vi "Meas Config Panel.vi"(8 "error in":errorcluster, 9 "force no GUI (False)":bool, 10 "always show setup (False)":bool, 11 "session in":T48={"adc"={"niScope"={"channel cfg"=[], "sessions"=[], "multi cards"=FALSE, "channels"=0, "type"=enum."n/a", "memory [B/chn]"=0, "ext. clock [Hz]"=0.0, "samples count"=0, "use streaming"=FALSE, "proc setup"={"packet size [smpl]"=0, "current timeout [s]"=0.0, "blk2blk timeout [s]"=0.0, "event time"=timestamp(0 s since 1904-01-01), "temp sampl T [s]"=0.0, "data queue"=refnum, "stop notifier"=refnum, "proc ref"=refnum}, "sample width [B]"=0, "ranges [V]"=[], "trigger setup"={"coupling"=1, "level [V]"=0.0, "slope"=0, "mode"=enum."Immediate"}, "fs [Hz]"=0.0, "bitres [bit]"=0}, "3458A"={"channels"=[], "sync unit"={"VISA"="", "type"=enum."Picotest U6200A"}, "awg unit"={"type"=enum."Agilent 331xxA to 332xxA", "VISA"="", "enable 10MHz ref"=FALSE}, "sync mode"=enum."MASTER-SLAVE, MASTER clocked by TIMER", "streaming mode"=FALSE, "idn mode"=enum."Auto", "sampling mode"=enum."DCV", "Ts [s]"=0.0, "sample memory [B]"=0, "proc setup"={"channel id"=0, "packet size [smpl]"=0, "current timeout [s]"=0.0, "blk2blk timeout [s]"=0.0, "event time"=timestamp(0 s since 1904-01-01), "stop notifier"=refnum, "data queues"=[], "proc refs"=[], "bus semaphore"=refnum}, "sample size [B]"=0, "sample count"=0, "aux data"={"channel id"=0, "valid?"=[], "gain [V]"=[], "timestamp [s]"=[], "Ts [s]"=0.0, "abs timestamp"=timestamp(0 s since 1904-01-01), "t [deg C]"=[]}, "ranges [V]"=[], "aperture [s]"=0.0, "LEVEL trigger"={"edge"=enum."POS", "level [V]"=0.0, "coupling"=enum."DC"}, "trigger mode"=enum."AUTO", "measure temp.?"=FALSE, "disp mesages"=[], "shared bus?"=FALSE, "disable display?"=FALSE, "aper mode"=enum."Manual", "aper rules"=[]}, "dsdll"={"dsdll"={"dsdll path"=path "", "dsdll handle"=[], "output devices"=[], "capture devices"=[]}, "channels"=0, "device id"=0, "channel idns"=[], "proc setup"={"packet size [smpl]"=0, "current timeout [s]"=0.0, "blk2blk timeout [s]"=0.0, "event time"=timestamp(0 s since 1904-01-01), "data queue"=refnum, "stop notifier"=refnum, "proc ref"=refnum}, "samples count"=0, "fs [Hz]"=0.0}, "type"=enum."niScope", "channel idn str"=[], "aux instr idn str"=[], "modified?"=FALSE, "simadc"={"channels"=[], "range [V]"=0.0, "Ts step [s]"=0.0, "time [s]"=0.0, "fs [Hz]"=0.0, "count"=0, "smpl offset"=0, "set count"=0, "bit res"=0}, "force rst?"=FALSE, "exit mode"=enum."Immediate reset", "exit dly"=0.0, "exit tmr"=timestamp(0 s since 1904-01-01), "busy?"=FALSE, "accessed?"=FALSE, "QuADC session"={"channel cfg"=[], "sessions"=[], "multi cards"=FALSE, "channels"=0, "type"=enum."n/a", "memory [B/chn]"=0, "ext. clock [Hz]"=0.0, "samples count"=0, "use streaming"=FALSE, "proc setup"={"packet size [smpl]"=0, "current timeout [s]"=0.0, "blk2blk timeout [s]"=0.0, "event time"=timestamp(0 s since 1904-01-01), "temp sampl T [s]"=0.0, "data queue"=refnum, "stop notifier"=refnum, "proc ref"=refnum}, "sample width [B]"=0, "ranges [V]"=[], "trigger setup"={"coupling"=1, "level [V]"=0.0, "slope"=0, "mode"=enum."Immediate"}, "fs [Hz]"=0.0, "bitres [bit]"=0}}, "sequence"=[], "sequence setup"={"group setups"=[], "average cycles"=0, "range mode"=enum."Keep defaults", "fs mode"=enum."Frequency", "rng even"=0.0, "rng odd"=0.0, "folder"=path "", "name base"="", "meas id"=0, "settle [s]"=0.0}, "golpi"=refnum, "processing setup"={"mode"=enum."Raw", "call after avgs?"=FALSE, "calculate?"=FALSE, "raw mode"={"command"="", "result mode"=enum."Display console output (only Octave)", "res variable"=""}, "QWTB"={"QWTB path"=path "", "alg filter path"="", "alg ids"=[], "alg parameters"=[], "parsed parameters"=[], "selected alg id"="", "selected unc mode"=enum."None", "qwtb mcc"=100, "qwtb timeout"=90, "qwtb covg"=95.0, "qwtb ofs"=0, "qwtb lim data"=0, "multicore"={"jobs folder"=path "", "cores"=0, "max jobs"=0, "mode"=enum."Singlecore"}, "unc once?"=FALSE}}, "corrections"={"transducers"={"channels"=[], "last path"=path ""}, "digitizer"={"last path"=path "", "channel paths"=[], "channel idns"=[], "correction name"="", "channel names"=[], "folders to copy"=[], "channel valid"=[], "correction path"=path "", "correction rel path"="", "rel folders to copy"=[]}}, "assist cfg"={"P"=0, "Q"=0, "rel shift"=0.0, "ref freq"=0.0, "min fs"=0.0, "max fs tol"=0.0, "min int"=0.0, "max int"=0.0, "max err"=0.0, "max timeout"=0.0}} {"corrections"."transducers"."channels"."Phase index" min=1 step=1; "adc"."QuADC session"."trigger setup"."level [V]" format="%.2f"; "adc"."QuADC session"."trigger setup"."coupling" items=["AC"=0, "DC"=1, "HF Reject"=3, "LF Reject"=4, "AC Plus HF Reject"=1001]; "adc"."QuADC session"."channel cfg"."Clock fr. (Hz)" min=0.0 format="%#_9p"; "adc"."QuADC session"."channel cfg"."Number of JJ" min=1; "adc"."QuADC session"."channel cfg"."Range [Vpk]" min=0.0; "adc"."QuADC session"."channel cfg"."Channel" min=0; "adc"."3458A"."channels"."Range [Vpk]" min=0.0; "adc"."niScope"."trigger setup"."level [V]" format="%.2f"; "adc"."niScope"."trigger setup"."coupling" items=["AC"=0, "DC"=1, "HF Reject"=3, "LF Reject"=4, "AC Plus HF Reject"=1001]; "adc"."niScope"."channel cfg"."Range [Vpk]" min=0.0; "adc"."niScope"."channel cfg"."Channel" min=0}) -> (0 "error out":errorcluster, 2 "canceled?":bool, 3 "session out":T48={"adc"={"niScope"={"channel cfg"=[], "sessions"=[], "multi cards"=FALSE, "channels"=0, "type"=enum."n/a", "memory [B/chn]"=0, "ext. clock [Hz]"=0.0, "samples count"=0, "use streaming"=FALSE, "proc setup"={"packet size [smpl]"=0, "current timeout [s]"=0.0, "blk2blk timeout [s]"=0.0, "event time"=timestamp(0 s since 1904-01-01), "temp sampl T [s]"=0.0, "data queue"=refnum, "stop notifier"=refnum, "proc ref"=refnum}, "sample width [B]"=0, "ranges [V]"=[], "trigger setup"={"coupling"=1, "level [V]"=0.0, "slope"=0, "mode"=enum."Immediate"}, "fs [Hz]"=0.0, "bitres [bit]"=0}, "3458A"={"channels"=[], "sync unit"={"VISA"="", "type"=enum."Picotest U6200A"}, "awg unit"={"type"=enum."Agilent 331xxA to 332xxA", "VISA"="", "enable 10MHz ref"=FALSE}, "sync mode"=enum."MASTER-SLAVE, MASTER clocked by TIMER", "streaming mode"=FALSE, "idn mode"=enum."Auto", "sampling mode"=enum."DCV", "Ts [s]"=0.0, "sample memory [B]"=0, "proc setup"={"channel id"=0, "packet size [smpl]"=0, "current timeout [s]"=0.0, "blk2blk timeout [s]"=0.0, "event time"=timestamp(0 s since 1904-01-01), "stop notifier"=refnum, "data queues"=[], "proc refs"=[], "bus semaphore"=refnum}, "sample size [B]"=0, "sample count"=0, "aux data"={"channel id"=0, "valid?"=[], "gain [V]"=[], "timestamp [s]"=[], "Ts [s]"=0.0, "abs timestamp"=timestamp(0 s since 1904-01-01), "t [deg C]"=[]}, "ranges [V]"=[], "aperture [s]"=0.0, "LEVEL trigger"={"edge"=enum."POS", "level [V]"=0.0, "coupling"=enum."DC"}, "trigger mode"=enum."AUTO", "measure temp.?"=FALSE, "disp mesages"=[], "shared bus?"=FALSE, "disable display?"=FALSE, "aper mode"=enum."Manual", "aper rules"=[]}, "dsdll"={"dsdll"={"dsdll path"=path "", "dsdll handle"=[], "output devices"=[], "capture devices"=[]}, "channels"=0, "device id"=0, "channel idns"=[], "proc setup"={"packet size [smpl]"=0, "current timeout [s]"=0.0, "blk2blk timeout [s]"=0.0, "event time"=timestamp(0 s since 1904-01-01), "data queue"=refnum, "stop notifier"=refnum, "proc ref"=refnum}, "samples count"=0, "fs [Hz]"=0.0}, "type"=enum."niScope", "channel idn str"=[], "aux instr idn str"=[], "modified?"=FALSE, "simadc"={"channels"=[], "range [V]"=0.0, "Ts step [s]"=0.0, "time [s]"=0.0, "fs [Hz]"=0.0, "count"=0, "smpl offset"=0, "set count"=0, "bit res"=0}, "force rst?"=FALSE, "exit mode"=enum."Immediate reset", "exit dly"=0.0, "exit tmr"=timestamp(0 s since 1904-01-01), "busy?"=FALSE, "accessed?"=FALSE, "QuADC session"={"channel cfg"=[], "sessions"=[], "multi cards"=FALSE, "channels"=0, "type"=enum."n/a", "memory [B/chn]"=0, "ext. clock [Hz]"=0.0, "samples count"=0, "use streaming"=FALSE, "proc setup"={"packet size [smpl]"=0, "current timeout [s]"=0.0, "blk2blk timeout [s]"=0.0, "event time"=timestamp(0 s since 1904-01-01), "temp sampl T [s]"=0.0, "data queue"=refnum, "stop notifier"=refnum, "proc ref"=refnum}, "sample width [B]"=0, "ranges [V]"=[], "trigger setup"={"coupling"=1, "level [V]"=0.0, "slope"=0, "mode"=enum."Immediate"}, "fs [Hz]"=0.0, "bitres [bit]"=0}}, "sequence"=[], "sequence setup"={"group setups"=[], "average cycles"=0, "range mode"=enum."Keep defaults", "fs mode"=enum."Frequency", "rng even"=0.0, "rng odd"=0.0, "folder"=path "", "name base"="", "meas id"=0, "settle [s]"=0.0}, "golpi"=refnum, "processing setup"={"mode"=enum."Raw", "call after avgs?"=FALSE, "calculate?"=FALSE, "raw mode"={"command"="", "result mode"=enum."Display console output (only Octave)", "res variable"=""}, "QWTB"={"QWTB path"=path "", "alg filter path"="", "alg ids"=[], "alg parameters"=[], "parsed parameters"=[], "selected alg id"="", "selected unc mode"=enum."None", "qwtb mcc"=100, "qwtb timeout"=90, "qwtb covg"=95.0, "qwtb ofs"=0, "qwtb lim data"=0, "multicore"={"jobs folder"=path "", "cores"=0, "max jobs"=0, "mode"=enum."Singlecore"}, "unc once?"=FALSE}}, "corrections"={"transducers"={"channels"=[], "last path"=path ""}, "digitizer"={"last path"=path "", "channel paths"=[], "channel idns"=[], "correction name"="", "channel names"=[], "folders to copy"=[], "channel valid"=[], "correction path"=path "", "correction rel path"="", "rel folders to copy"=[]}}, "assist cfg"={"P"=0, "Q"=0, "rel shift"=0.0, "ref freq"=0.0, "min fs"=0.0, "max fs tol"=0.0, "min int"=0.0, "max int"=0.0, "max err"=0.0, "max timeout"=0.0}} {"corrections"."transducers"."channels"."Phase index" min=1 step=1; "adc"."QuADC session"."trigger setup"."level [V]" format="%.2f"; "adc"."QuADC session"."trigger setup"."coupling" items=["AC"=0, "DC"=1, "HF Reject"=3, "LF Reject"=4, "AC Plus HF Reject"=1001]; "adc"."QuADC session"."channel cfg"."Clock fr. (Hz)" min=0.0 format="%#_9p"; "adc"."QuADC session"."channel cfg"."Number of JJ" min=1; "adc"."QuADC session"."channel cfg"."Range [Vpk]" min=0.0; "adc"."QuADC session"."channel cfg"."Channel" min=0; "adc"."3458A"."channels"."Range [Vpk]" min=0.0; "adc"."niScope"."trigger setup"."level [V]" format="%.2f"; "adc"."niScope"."trigger setup"."coupling" items=["AC"=0, "DC"=1, "HF Reject"=3, "LF Reject"=4, "AC Plus HF Reject"=1001]; "adc"."niScope"."channel cfg"."Range [Vpk]" min=0.0; "adc"."niScope"."channel cfg"."Channel" min=0})   [LabVIEW 2013]
doc: "New measurement configuration panel."
uses:
  Meas Session.ctl
  adc/ADC Session.ctl
  drivers/niScope/niScope Session.ctl
  drivers/niScope/niScope Virtual Channel Config.ctl
  drivers/niScope/niScope Virtual Channel Mode.ctl
  drivers/niScope/niScope Virtual Channel Input Z.ctl
  drivers/niScope/niScope Virtual Channel Coupling.ctl
  drivers/niScope/niScope Type.ctl
  drivers/niScope/niScope Digitizing Process Options.ctl
  drivers/niScope/niScope Data Packet.ctl
  drivers/niScope/niScope Trigger Setup.ctl
  <instrlib>/niScope/Controls/niScope trigger coupling.ctl
  <instrlib>/niScope/Controls/niScope trigger slope.ctl
  drivers/DMM/3458A Digitizer Session.ctl
  drivers/DMM/3458A Virtual Channel Config.ctl
  drivers/Counter/Counter Session.ctl
  drivers/Counter/Counter Type.ctl
  drivers/AWG/AWG Session.ctl
  drivers/AWG/AWG Type.ctl
  drivers/DMM/3458A Sync Mode.ctl
  drivers/DMM/3458A Idn Mode.ctl
  drivers/DMM/3458A Digitizing Low Levels/Configure/Sampling Mode.ctl
  drivers/DMM/3458A Digitizing Process Options.ctl
  drivers/DMM/3458A Data Packet.ctl
  drivers/DMM/3458A Aux Record Data.ctl
  drivers/DMM/3458A Digitizing Low Levels/Configure/Level Setup.ctl
  drivers/DMM/3458A Digitizing Low Levels/Configure/First Sample Trigger.ctl
  drivers/DMM/3458A Aperture Selection Mode.ctl
  drivers/dsdll/DSDLL Session.ctl
  drivers/dsdll/dsdll.lvlibp/dsdll_instance.ctl
  drivers/dsdll/dsdll.lvlibp/dsdll_device_record.ctl
  drivers/dsdll/DSDLL Process Config.ctl
  drivers/dsdll/DSDLL Data Packet.ctl
  adc/ADC Type.ctl
  drivers/simulated_adc/SimAdc Config.ctl
  drivers/simulated_adc/SimAdc Channel Cfg.ctl
  adc/ADC On Close Action.ctl
  drivers/Quatsch_driver/QuADCDriver/QuADC Session.ctl
  drivers/Quatsch_driver/QuADCDriver/QuADC Virtual Channel Config.ctl
  drivers/Quatsch_driver/QuADCDriver/QuADC Virtual Channel Mode.ctl
  drivers/Quatsch_driver/QuADCDriver/QuADC Virtual Channel Input Z.ctl
  drivers/Quatsch_driver/QuADCDriver/QuADC Virtual Channel Coupling.ctl
  drivers/Quatsch_driver/QuADCDriver/QuADC Type.ctl
  drivers/Quatsch_driver/QuADCDriver/QuADC Digitizing Process Options.ctl
  drivers/Quatsch_driver/QuADCDriver/QuADC Data Packet.ctl
  drivers/Quatsch_driver/QuADCDriver/QuADC Trigger Setup.ctl
  Meas Sequence Item.ctl
  Meas Sampling Configuration.ctl
  adc/ADC Trig Config.ctl
  adc/ADC Trig Mode Source.ctl
  adc/ADC Trig Coupling.ctl
  adc/ADC Trig Slope.ctl
  processing/QWTB/Meas Proc QWTB Algorithm Parameter Data.ctl
  Meas Sequence Configuration.ctl
  Meas Range Mode.ctl
  Meas Sampling Rate Mode.ctl
  octave/golpi/mpc/golpi_session_ref.ctl
  octave/golpi/mpc/golpi_session.ctl
  octave/golpi/GOLPI Library.lvlibp/Public/GOLPI reference Type Def.ctl
  octave/golpi/GOLPI Library.lvlibp/LV Process source distribution/Pipe Handle.ctl
  processing/Meas Process Config.ctl
  processing/Meas Process Mode.ctl
  processing/Meas Process Raw Config.ctl
  processing/Meas Process Raw Result Mode.ctl
  processing/QWTB/Meas Proc QWTB Setup.ctl
  processing/QWTB/Meas Proc QWTB Uncertainty Mode.ctl
  processing/QWTB/Meas Proc QWTB Multicore Setup.ctl
  processing/QWTB/Meas Proc QWTB Multicore Type.ctl
  Corrections/Corr Setup.ctl
  Corrections/Corr Tranducer Item.ctl
  Corrections/Corr Digitizers.ctl
  Assist/Assist Panel Setup.ctl
  varilib/SGUI Assign References Mode.ctl
  other/GUI Panel Control Action.ctl
  adc/ADC Capabilities Parameters.ctl
  varilib/SGUI Set Multiple Reals By Label.vi
  varilib/SGUI Set Single Real By Label.vi
  varilib/SGUI Set Single Integer By Label.vi
  varilib/varilib.lvlib
  drivers/niScope/niScope Virtual Digitizer.lvlib
  drivers/DMM/3458A Virtual Digitizer.lvlib
  drivers/Counter/Counter.lvlib
  drivers/AWG/AWG.lvlib
  drivers/DMM/3458A Digitizing Low Levels/3458A Digitizing Low Levels.lvlib
  drivers/dsdll/dsdll.lvlibp
  drivers/dsdll/DSDLL Virtual Digitizer.lvlib
  octave/golpi/GOLPI Library.lvlibp/LV Process source distribution/LV Process library.lvlib
  octave/golpi/GOLPI Library.lvlibp
  octave/golpi/mpc/GOLPI Multi Process.lvlib
  drivers/Quatsch_driver/QuADCDriver/QuADC Virtual Digitizer.lvlib
panel:
  in  "rep delay":dbl caption="Repetition settling [s]"
  in  "btn assist":bool
  in  "smpl time":dbl caption="Meas. time [s]"
  out "smpl time max":dbl caption="Max. time [s]" format="%#_6p"
  out "meas full":path caption="Full measurement base path preview"
  in  "meas id":i32 caption="Measurement number" min=0 max=9999 step=1
  in  "btn proc":bool
  in  "calc result?":bool caption="Enable result calculation?"
  in  "meas name":string caption="Measurement name base"
  in  "data folder":path caption="Folder for measurements data files"
  in  "avg cycles":i32=1 caption="Repetition cycles"
  in  "range even":dbl
  in  "range odd":dbl caption="All ranges [V]"
  in  "range mode":T1 caption="Voltage range selection"
  out "smpl count max":dbl caption="Max. samples count" format="%#_6p"
  in  "smpl count":i64 caption="Samples count"
  out "aperture max":dbl caption="smpl rate min" format="%#_5p"
  out "aperture min":dbl caption="Aperture range [s]" format="%#_5p"
  out "smpl rate max":dbl caption="smpl rate min" format="%#_5p"
  out "smpl rate min":dbl caption="Sampling period range [s]" format="%#_5p"
  in  "trig coupling":T2 caption="Trigger coupling"
  in  "trig slope":T3 caption="Trigger slope"
  in  "trig level":dbl caption="Level [V]" format="%#_3p"
  in  "trig mode":T4 caption="Trigger mode"
  in  "aperture":dbl caption="Aperture [s]" format="%#_3p"
  out "adc":T5={"niScope"={"channel cfg"=[], "sessions"=[], "multi cards"=FALSE, "channels"=0, "type"=enum."n/a", "memory [B/chn]"=0, "ext. clock [Hz]"=0.0, "samples count"=0, "use streaming"=FALSE, "proc setup"={"packet size [smpl]"=0, "current timeout [s]"=0.0, "blk2blk timeout [s]"=0.0, "event time"=timestamp(0 s since 1904-01-01), "temp sampl T [s]"=0.0, "data queue"=refnum, "stop notifier"=refnum, "proc ref"=refnum}, "sample width [B]"=0, "ranges [V]"=[], "trigger setup"={"coupling"=1, "level [V]"=0.0, "slope"=0, "mode"=enum."Immediate"}, "fs [Hz]"=0.0, "bitres [bit]"=0}, "3458A"={"channels"=[], "sync unit"={"VISA"="", "type"=enum."Picotest U6200A"}, "awg unit"={"type"=enum."Agilent 331xxA to 332xxA", "VISA"="", "enable 10MHz ref"=FALSE}, "sync mode"=enum."MASTER-SLAVE, MASTER clocked by TIMER", "streaming mode"=FALSE, "idn mode"=enum."Auto", "sampling mode"=enum."DCV", "Ts [s]"=0.0, "sample memory [B]"=0, "proc setup"={"channel id"=0, "packet size [smpl]"=0, "current timeout [s]"=0.0, "blk2blk timeout [s]"=0.0, "event time"=timestamp(0 s since 1904-01-01), "stop notifier"=refnum, "data queues"=[], "proc refs"=[], "bus semaphore"=refnum}, "sample size [B]"=0, "sample count"=0, "aux data"={"channel id"=0, "valid?"=[], "gain [V]"=[], "timestamp [s]"=[], "Ts [s]"=0.0, "abs timestamp"=timestamp(0 s since 1904-01-01), "t [deg C]"=[]}, "ranges [V]"=[], "aperture [s]"=0.0, "LEVEL trigger"={"edge"=enum."POS", "level [V]"=0.0, "coupling"=enum."DC"}, "trigger mode"=enum."AUTO", "measure temp.?"=FALSE, "disp mesages"=[], "shared bus?"=FALSE, "disable display?"=FALSE, "aper mode"=enum."Manual", "aper rules"=[]}, "dsdll"={"dsdll"={"dsdll path"=path "", "dsdll handle"=[], "output devices"=[], "capture devices"=[]}, "channels"=0, "device id"=0, "channel idns"=[], "proc setup"={"packet size [smpl]"=0, "current timeout [s]"=0.0, "blk2blk timeout [s]"=0.0, "event time"=timestamp(0 s since 1904-01-01), "data queue"=refnum, "stop notifier"=refnum, "proc ref"=refnum}, "samples count"=0, "fs [Hz]"=0.0}, "type"=enum."niScope", "channel idn str"=[], "aux instr idn str"=[], "modified?"=FALSE, "simadc"={"channels"=[], "range [V]"=0.0, "Ts step [s]"=0.0, "time [s]"=0.0, "fs [Hz]"=0.0, "count"=0, "smpl offset"=0, "set count"=0, "bit res"=0}, "force rst?"=FALSE, "exit mode"=enum."Immediate reset", "exit dly"=0.0, "exit tmr"=timestamp(0 s since 1904-01-01), "busy?"=FALSE, "accessed?"=FALSE, "QuADC session"={"channel cfg"=[], "sessions"=[], "multi cards"=FALSE, "channels"=0, "type"=enum."n/a", "memory [B/chn]"=0, "ext. clock [Hz]"=0.0, "samples count"=0, "use streaming"=FALSE, "proc setup"={"packet size [smpl]"=0, "current timeout [s]"=0.0, "blk2blk timeout [s]"=0.0, "event time"=timestamp(0 s since 1904-01-01), "temp sampl T [s]"=0.0, "data queue"=refnum, "stop notifier"=refnum, "proc ref"=refnum}, "sample width [B]"=0, "ranges [V]"=[], "trigger setup"={"coupling"=1, "level [V]"=0.0, "slope"=0, "mode"=enum."Immediate"}, "fs [Hz]"=0.0, "bitres [bit]"=0}} {"QuADC session"."trigger setup"."level [V]" format="%.2f"; "QuADC session"."trigger setup"."coupling" items=["AC"=0, "DC"=1, "HF Reject"=3, "LF Reject"=4, "AC Plus HF Reject"=1001]; "QuADC session"."channel cfg"."Clock fr. (Hz)" min=0.0 format="%#_9p"; "QuADC session"."channel cfg"."Number of JJ" min=1; "QuADC session"."channel cfg"."Range [Vpk]" min=0.0; "QuADC session"."channel cfg"."Channel" min=0; "3458A"."channels"."Range [Vpk]" min=0.0; "niScope"."trigger setup"."level [V]" format="%.2f"; "niScope"."trigger setup"."coupling" items=["AC"=0, "DC"=1, "HF Reject"=3, "LF Reject"=4, "AC Plus HF Reject"=1001]; "niScope"."channel cfg"."Range [Vpk]" min=0.0; "niScope"."channel cfg"."Channel" min=0}
  in  "btn cancel":bool
  in  "btn ok":bool
  in  "fs mode":T47 caption="Sampling rate mode"
  in  "smpl rate":dbl caption="Sampling period [s]"
  # "Use following variables in the name base:\n  %id% - measurement number in format DDDD\n  %date% - date of the measurement YYYYMMDD\n  %time% - time of the measurement HH-MM-SS\nExample:\n  my_measurement_%id%"
  # "IP Address"
  # "."
  # "."
  # "."
  # ":"
  # "ADC:"
  # "IP Address"
  # "."
  # "."
  # "."
  # ":"
  # "ADC:"
  # "IP Address"
  # "."
  # "."
  # "."
  # ":"
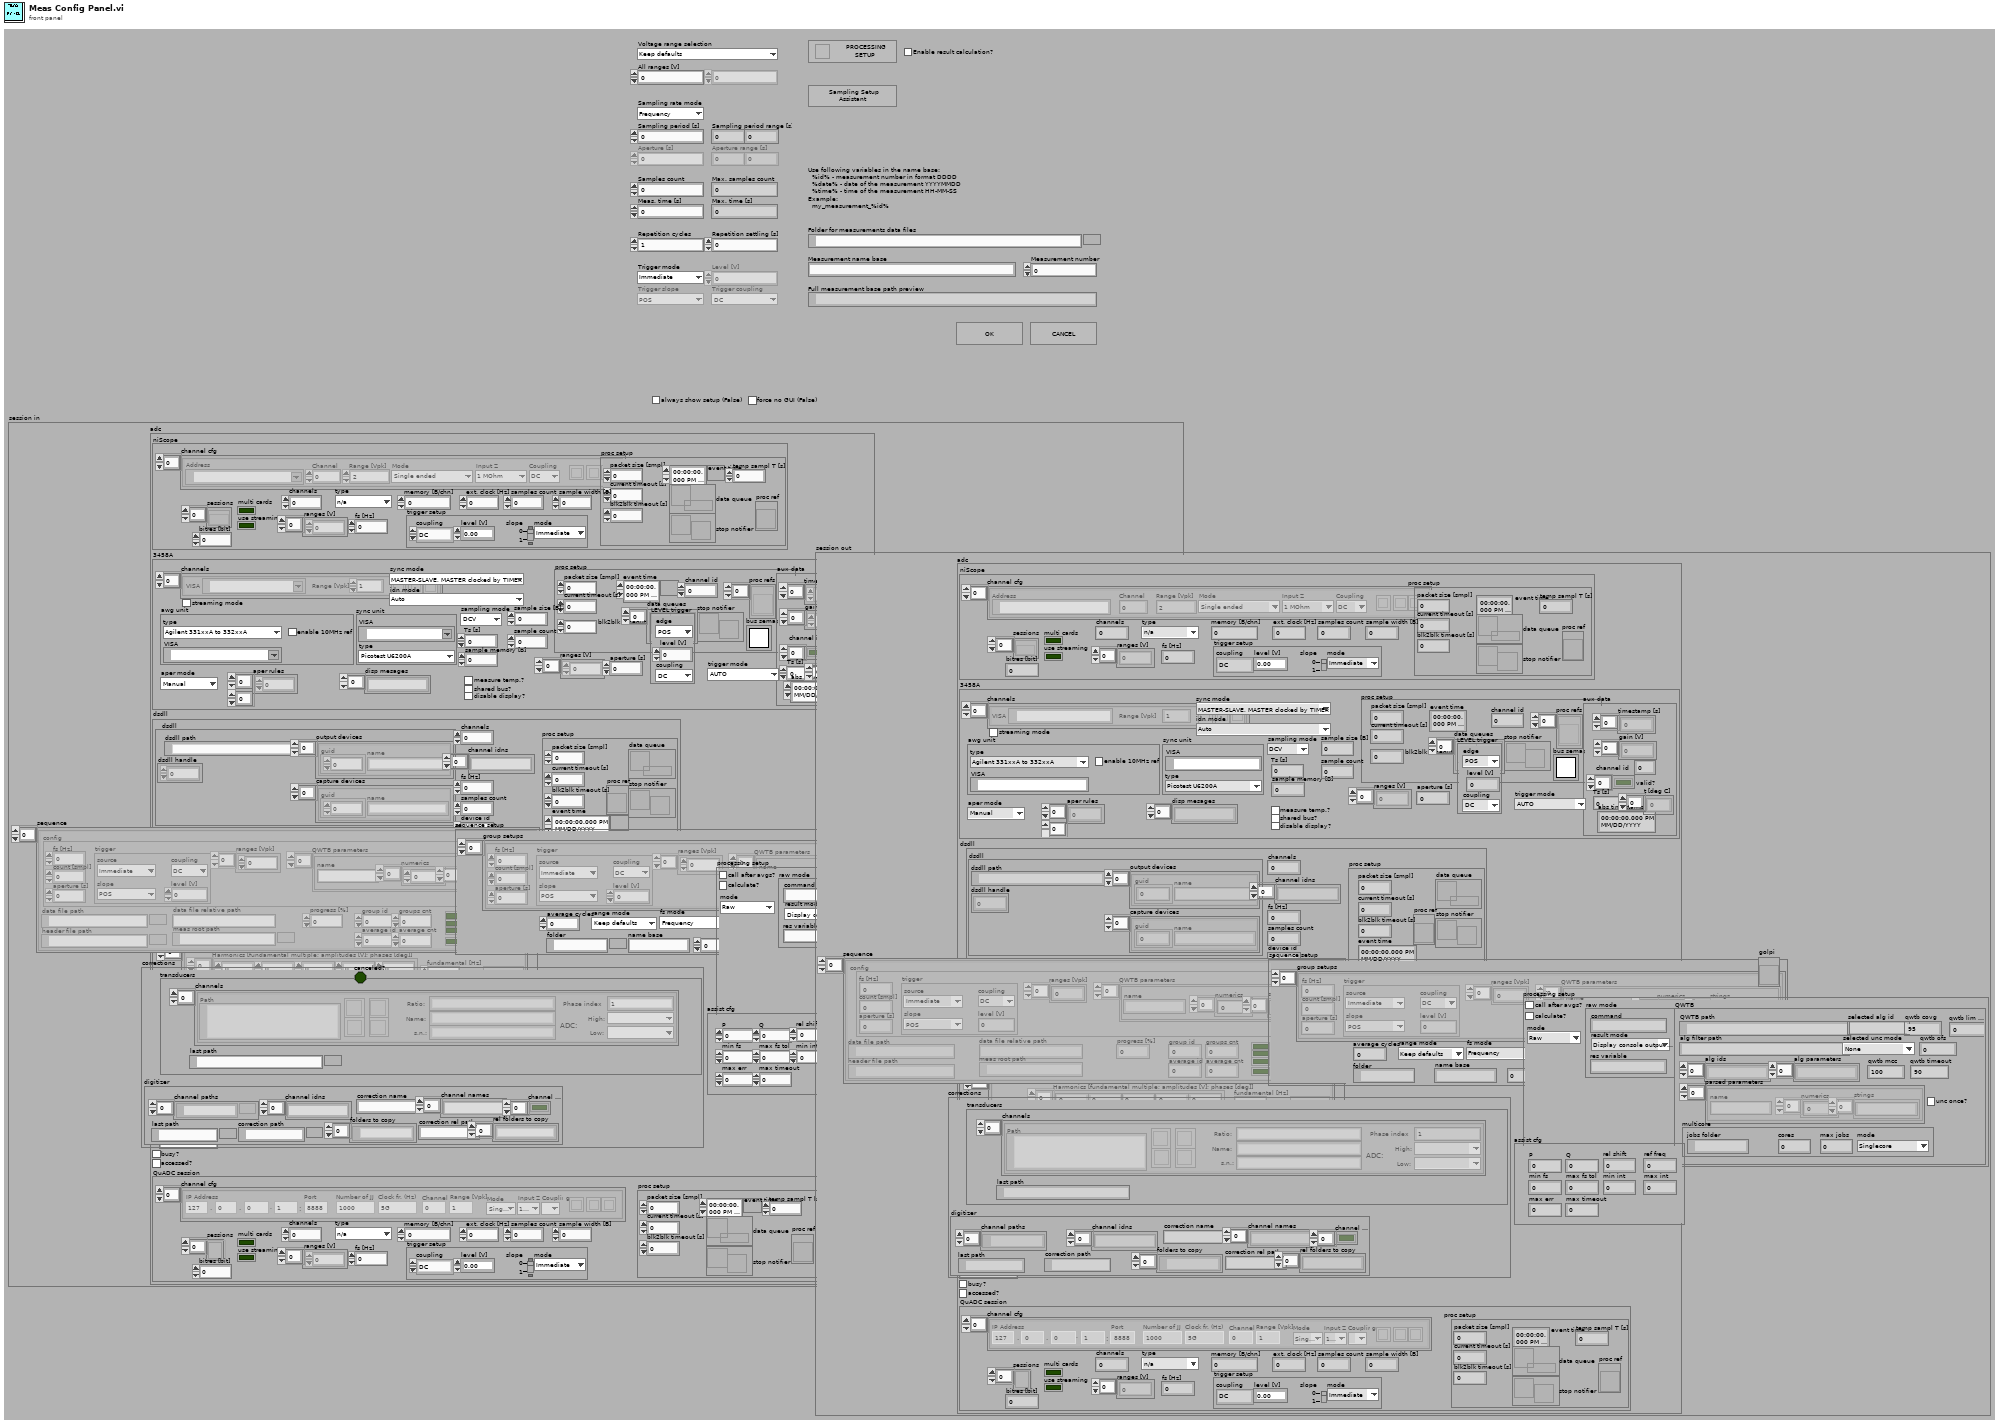
[diagram p1: front panel]
types:
  T1 = typedef "Meas Range Mode.ctl" = enum16{"Keep defaults", "Set All channels", "Set Odd and Even channels"}
  T2 = typedef "ADC Trig Coupling.ctl" = enum16{"DC", "AC"}
  T3 = typedef "ADC Trig Slope.ctl" = enum16{"POS", "NEG"}
  T4 = typedef "ADC Trig Mode Source.ctl" = enum16{"Immediate", "External", "Level"}
  T5 = typedef "ADC Session.ctl" = cluster{"niScope":T6, "3458A":T16, "dsdll":T31, "type":T35, "channel idn str":string[], "aux instr idn str":string[], "modified?":bool, "simadc":T36, "force rst?":bool, "exit mode":T38, "exit dly":dbl, "exit tmr":timestamp, "busy?":bool, "accessed?":bool, "QuADC session":T39}
  T6 = typedef "niScope Virtual Digitizer.lvlib/niScope Session.ctl" = cluster{"channel cfg":T7[], "sessions":refnum<k20>[], "multi cards":bool, "channels":i32, "type":T11, "memory [B/chn]":i32, "ext. clock [Hz]":dbl, "samples count":i64, "use streaming":bool, "proc setup":T12, "sample width [B]":i32, "ranges [V]":dbl[], "trigger setup":T13, "fs [Hz]":dbl, "bitres [bit]":i32}
  T7 = typedef "niScope Virtual Digitizer.lvlib/niScope Virtual Channel Config.ctl" = cluster{"Address":refnum<k15>, "Channel":i32, "Mode":T8, "Input Z":T9, "Coupling":T10, "Range [Vpk]":dbl, "btn clr":bool, "btn up":bool, "btn down":bool}
  T8 = typedef "niScope Virtual Digitizer.lvlib/niScope Virtual Channel Mode.ctl" = enum16{"Single ended", "Unbal. differential", "Differential"}
  T9 = typedef "niScope Virtual Digitizer.lvlib/niScope Virtual Channel Input Z.ctl" = enum16{"1 MOhm", "50 Ohm"}
  T10 = typedef "niScope Virtual Digitizer.lvlib/niScope Virtual Channel Coupling.ctl" = enum16{"AC", "DC", "GND"}
  T11 = typedef "niScope Virtual Digitizer.lvlib/niScope Type.ctl" = enum16{"n/a", "5922"}
  T12 = typedef "niScope Virtual Digitizer.lvlib/niScope Digitizing Process Options.ctl" = cluster{"packet size [smpl]":i64, "current timeout [s]":dbl, "blk2blk timeout [s]":dbl, "event time":timestamp, "temp sampl T [s]":dbl, "data queue":refnum<queue>, "stop notifier":refnum<notifier>, "proc ref":refnum<vi>}
  T13 = typedef "niScope Virtual Digitizer.lvlib/niScope Trigger Setup.ctl" = cluster{"coupling":T14, "level [V]":dbl, "slope":T15, "mode":enum16{"Immediate", "External", "Level"}}
  T14 = typedef "niScope trigger coupling.ctl" = u16
  T15 = typedef "niScope trigger slope.ctl" = i32
  T16 = typedef "3458A Virtual Digitizer.lvlib/3458A Digitizer Session.ctl" = cluster{"channels":T17[], "sync unit":T18, "awg unit":T20, "sync mode":T22, "streaming mode":bool, "idn mode":T23, "sampling mode":T24, "Ts [s]":dbl, "sample memory [B]":i32, "proc setup":T25, "sample size [B]":i32, "sample count":i32, "aux data":T27, "ranges [V]":dbl[], "aperture [s]":dbl, "LEVEL trigger":T28, "trigger mode":T29, "measure temp.?":bool, "disp mesages":string[], "shared bus?":bool, "disable display?":bool, "aper mode":T30, "aper rules":dbl[][]}
  T17 = typedef "3458A Virtual Digitizer.lvlib/3458A Virtual Channel Config.ctl" = cluster{"VISA":refnum<visa-resource-name>, "Range [Vpk]":dbl, "btn clr":bool, "btn up":bool, "btn down":bool}
  T18 = typedef "Counter.lvlib/Counter Session.ctl" = cluster{"VISA":refnum<visa-resource-name>, "type":T19}
  T19 = typedef "Counter.lvlib/Counter Type.ctl" = enum16{"Picotest U6200A", "dummy"}
  T20 = typedef "AWG.lvlib/AWG Session.ctl" = cluster{"type":T21, "VISA":refnum<visa-resource-name>, "enable 10MHz ref":bool}
  T21 = typedef "AWG.lvlib/AWG Type.ctl" = enum16{"Agilent 331xxA to 332xxA", "Agilent 335xxA to 336xxA", "Tektronix AFG3101C", "dummy"}
  T22 = typedef "3458A Virtual Digitizer.lvlib/3458A Sync Mode.ctl" = enum16{"MASTER-SLAVE, MASTER clocked by TIMER", "MASTER-SLAVE, MASTER clocked by AWG", "ALL clocked by AWG", "MASTER-SLAVE, ALL clocked by TIMER", "ALL clocked by AWG with DFLL"}
  T23 = typedef "3458A Virtual Digitizer.lvlib/3458A Idn Mode.ctl" = enum16{"Auto", "Sequential (chn A, chn B, ...)", "From calibration string"}
  T24 = typedef "3458A Virtual Digitizer.lvlib/3458A Digitizing Low Levels.lvlib/Sampling Mode.ctl" = enum16{"DCV", "DSDC", "DSAC"}
  T25 = typedef "3458A Virtual Digitizer.lvlib/3458A Digitizing Process Options.ctl" = cluster{"channel id":i32, "packet size [smpl]":i32, "current timeout [s]":dbl, "blk2blk timeout [s]":dbl, "event time":timestamp, "stop notifier":refnum<notifier>, "data queues":refnum<queue>[], "proc refs":refnum<vi>[], "bus semaphore":T26}
  T26 = typedef "Semaphore RefNum" = refnum<k1>
  T27 = typedef "3458A Virtual Digitizer.lvlib/3458A Aux Record Data.ctl" = cluster{"channel id":i32, "valid?":bool[], "gain [V]":dbl[], "timestamp [s]":dbl[], "Ts [s]":dbl, "abs timestamp":timestamp, "t [deg C]":dbl[]}
  T28 = typedef "3458A Virtual Digitizer.lvlib/3458A Digitizing Low Levels.lvlib/Level Setup.ctl" = cluster{"edge":enum16{"POS", "NEG"}, "level [V]":dbl, "coupling":enum16{"DC", "AC"}}
  T29 = typedef "3458A Virtual Digitizer.lvlib/3458A Digitizing Low Levels.lvlib/First Sample Trigger.ctl" = enum16{"AUTO", "EXT", "SYN", "SGL", "HOLD", "LEVEL"}
  T30 = typedef "3458A Virtual Digitizer.lvlib/3458A Aperture Selection Mode.ctl" = enum16{"Manual", "Maximum", "Table"}
  T31 = typedef "DSDLL Virtual Digitizer.lvlib/DSDLL Session.ctl" = cluster{"dsdll":T32, "channels":i32, "device id":i32, "channel idns":string[], "proc setup":T34, "samples count":i32, "fs [Hz]":dbl}
  T32 = typedef "dsdll.lvlibp/dsdll_instance.ctl" = cluster{"dsdll path":path, "dsdll handle":u8[], "output devices":T33[], "capture devices":T33[]}
  T33 = typedef "dsdll.lvlibp/dsdll_device_record.ctl" = cluster{"guid":u8[], "name":string}
  T34 = typedef "DSDLL Virtual Digitizer.lvlib/DSDLL Process Config.ctl" = cluster{"packet size [smpl]":i32, "current timeout [s]":dbl, "blk2blk timeout [s]":dbl, "event time":timestamp, "data queue":refnum<queue>, "stop notifier":refnum<notifier>, "proc ref":refnum<vi>}
  T35 = typedef "ADC Type.ctl" = enum16{"niScope", "3458A", "DirectSound DLL", "dummy", "QuADC"}
  T36 = typedef "SimAdc Config.ctl" = cluster{"channels":T37[], "range [V]":dbl, "Ts step [s]":dbl, "time [s]":dbl, "fs [Hz]":dbl, "count":i64, "smpl offset":i64, "set count":i64, "bit res":i32}
  T37 = typedef "SimAdc Channel Cfg.ctl" = cluster{"harmonics":dbl[][], "btn clear":bool, "noise":dbl, "fundamental [Hz]":dbl}
  T38 = typedef "ADC On Close Action.ctl" = enum16{"Immediate reset", "Delayed reset"}
  T39 = typedef "QuADC Virtual Digitizer.lvlib/QuADC Session.ctl" = cluster{"channel cfg":T40[], "sessions":refnum<k5>[], "multi cards":bool, "channels":i32, "type":T44, "memory [B/chn]":i32, "ext. clock [Hz]":dbl, "samples count":i64, "use streaming":bool, "proc setup":T45, "sample width [B]":i32, "ranges [V]":dbl[], "trigger setup":T46, "fs [Hz]":dbl, "bitres [bit]":i32}
  T40 = typedef "QuADC Virtual Digitizer.lvlib/QuADC Virtual Channel Config.ctl" = cluster{"Channel":i32, "Mode":T41, "Input Z":T42, "Coupling":T43, "Range [Vpk]":dbl, "btn clr":bool, "btn up":bool, "btn down":bool, "IP address A":u8, "IP address B":u8, "IP address C":u8, "IP address D":u8, "Port":u16, "Number of JJ":u32, "Clock fr. (Hz)":dbl}
  T41 = typedef "QuADC Virtual Digitizer.lvlib/QuADC Virtual Channel Mode.ctl" = enum16{"Single ended", "Unbal. differential", "Differential"}
  T42 = typedef "QuADC Virtual Digitizer.lvlib/QuADC Virtual Channel Input Z.ctl" = enum16{"1 MOhm", "50 Ohm"}
  T43 = typedef "QuADC Virtual Digitizer.lvlib/QuADC Virtual Channel Coupling.ctl" = enum16{"AC", "DC", "GND"}
  T44 = typedef "QuADC Virtual Digitizer.lvlib/QuADC Type.ctl" = enum16{"n/a", "v1"}
  T45 = typedef "QuADC Virtual Digitizer.lvlib/QuADC Digitizing Process Options.ctl" = cluster{"packet size [smpl]":i64, "current timeout [s]":dbl, "blk2blk timeout [s]":dbl, "event time":timestamp, "temp sampl T [s]":dbl, "data queue":refnum<queue>, "stop notifier":refnum<notifier>, "proc ref":refnum<vi>}
  T46 = typedef "QuADC Virtual Digitizer.lvlib/QuADC Trigger Setup.ctl" = cluster{"coupling":T14, "level [V]":dbl, "slope":T15, "mode":enum16{"Immediate", "External", "Level"}}
  T47 = typedef "Meas Sampling Rate Mode.ctl" = enum16{"Frequency", "Period"}
  T48 = typedef "Meas Session.ctl" = cluster{"adc":T5, "sequence":T49[], "sequence setup":T53, "golpi":T54, "processing setup":T55, "corrections":T63, "assist cfg":T66}
  T49 = typedef "Meas Sequence Item.ctl" = cluster{"config":T50, "data file path":path, "header file path":path, "group id":i32, "average id":i32, "group done?":bool, "adc modified?":bool, "source modified?":bool, "progress [%]":dbl, "groups cnt":i32, "average cnt":i32, "data file relative path":string, "meas root path":path, "calculate?":bool}
  T50 = typedef "Meas Sampling Configuration.ctl" = cluster{"fs [Hz]":dbl, "count [smpl]":i64, "aperture [s]":dbl, "trigger":T51, "ranges [Vpk]":dbl[], "QWTB parameters":T52[]}
  T51 = typedef "ADC Trig Config.ctl" = cluster{"source":T4, "level [V]":dbl, "coupling":T2, "slope":T3}
  T52 = typedef "Meas Proc QWTB Algorithm Parameter Data.ctl" = cluster{"name":string, "numerics":dbl[], "strings":string[]}
  T53 = typedef "Meas Sequence Configuration.ctl" = cluster{"group setups":T50[], "average cycles":i32, "range mode":T1, "fs mode":T47, "rng even":dbl, "rng odd":dbl, "folder":path, "name base":string, "meas id":i32, "settle [s]":dbl}
  T54 = typedef "GOLPI Multi Process.lvlib/golpi_session_ref.ctl" = refnum<vi>
  T55 = typedef "Meas Process Config.ctl" = cluster{"mode":T56, "call after avgs?":bool, "calculate?":bool, "raw mode":T57, "QWTB":T59}
  T56 = typedef "Meas Process Mode.ctl" = enum16{"Raw", "QWTB"}
  T57 = typedef "Meas Process Raw Config.ctl" = cluster{"command":string, "result mode":T58, "res variable":string}
  T58 = typedef "Meas Process Raw Result Mode.ctl" = enum16{"Display console output (only Octave)", "Display string variable", "Display result file %respath%"}
  T59 = typedef "Meas Proc QWTB Setup.ctl" = cluster{"QWTB path":path, "alg filter path":string, "alg ids":string[], "alg parameters":string[], "parsed parameters":T52[], "selected alg id":string, "selected unc mode":T60, "qwtb mcc":i32, "qwtb timeout":i32, "qwtb covg":dbl, "qwtb ofs":i64, "qwtb lim data":i64, "multicore":T61, "unc once?":bool}
  T60 = typedef "Meas Proc QWTB Uncertainty Mode.ctl" = enum16{"None", "GUF", "Monte Carlo"}
  T61 = typedef "Meas Proc QWTB Multicore Setup.ctl" = cluster{"jobs folder":path, "cores":i32, "max jobs":i32, "mode":T62}
  T62 = typedef "Meas Proc QWTB Multicore Type.ctl" = enum16{"Singlecore", "Multicore", "Multistation"}
  T63 = typedef "Corr Setup.ctl" = cluster{"transducers":cluster{"channels":T64[], "last path":path}, "digitizer":T65}
  T64 = typedef "Corr Tranducer Item.ctl" = cluster{"Path":path, "Ratio:":string, "Name:":string, "btn rem":bool, "btn up":bool, "btn down":bool, "s.n.:":string, "btn open":bool, "ratio o/i":dbl, "chn hi":u16, "chn lo":u16, "Phase index":i32}
  T65 = typedef "Corr Digitizers.ctl" = cluster{"last path":path, "channel paths":path[], "channel idns":string[], "correction name":string, "channel names":string[], "folders to copy":path[], "channel valid":bool[], "correction path":path, "correction rel path":string, "rel folders to copy":string[]}
  T66 = typedef "Assist Panel Setup.ctl" = cluster{"P":i32, "Q":i32, "rel shift":dbl, "ref freq":dbl, "min fs":dbl, "max fs tol":dbl, "min int":dbl, "max int":dbl, "max err":dbl, "max timeout":dbl}
  T67 = typedef "GUI Panel Control Action.ctl" = enum16{"Open panel", "Close panel", "Bring To Front"}
  T68 = typedef "varilib.lvlib/SGUI Assign References Mode.ctl" = enum16{"Add to stack", "Overwrite", "Release last", "Release ID"}
  T69 = typedef "ADC Capabilities Parameters.ctl" = cluster{"fs [Hz]":dbl, "aperture [s]":dbl}
  T70 = typedef "ADC Capabilities.ctl" = cluster{"max samples count":i64, "max fs [Hz]":ext, "min fs [Hz]":ext, "Ts step [s]":ext, "max Ts [s]":ext, "min Ts [s]":ext, "allows streaming?":bool, "streaming on?":bool, "has level trig?":bool, "has ext trig?":bool, "has aperture?":bool, "aper min [s]":dbl, "aper max [s]":dbl, "channels count":i32, "has ranges?":bool, "has temperature?":bool, "has temperature log?":bool, "has selfcal?":bool, "fs step [Hz]":ext, "smpl rate step mode":T71}
  T71 = typedef "ADC Sampling Rate Step Mode.ctl" = enum16{"const period", "const frequency"}
  T72 = typedef "Assist Sampling Setup.ctl" = cluster{"fs [Hz]":ext, "N":i64, "error":dbl}
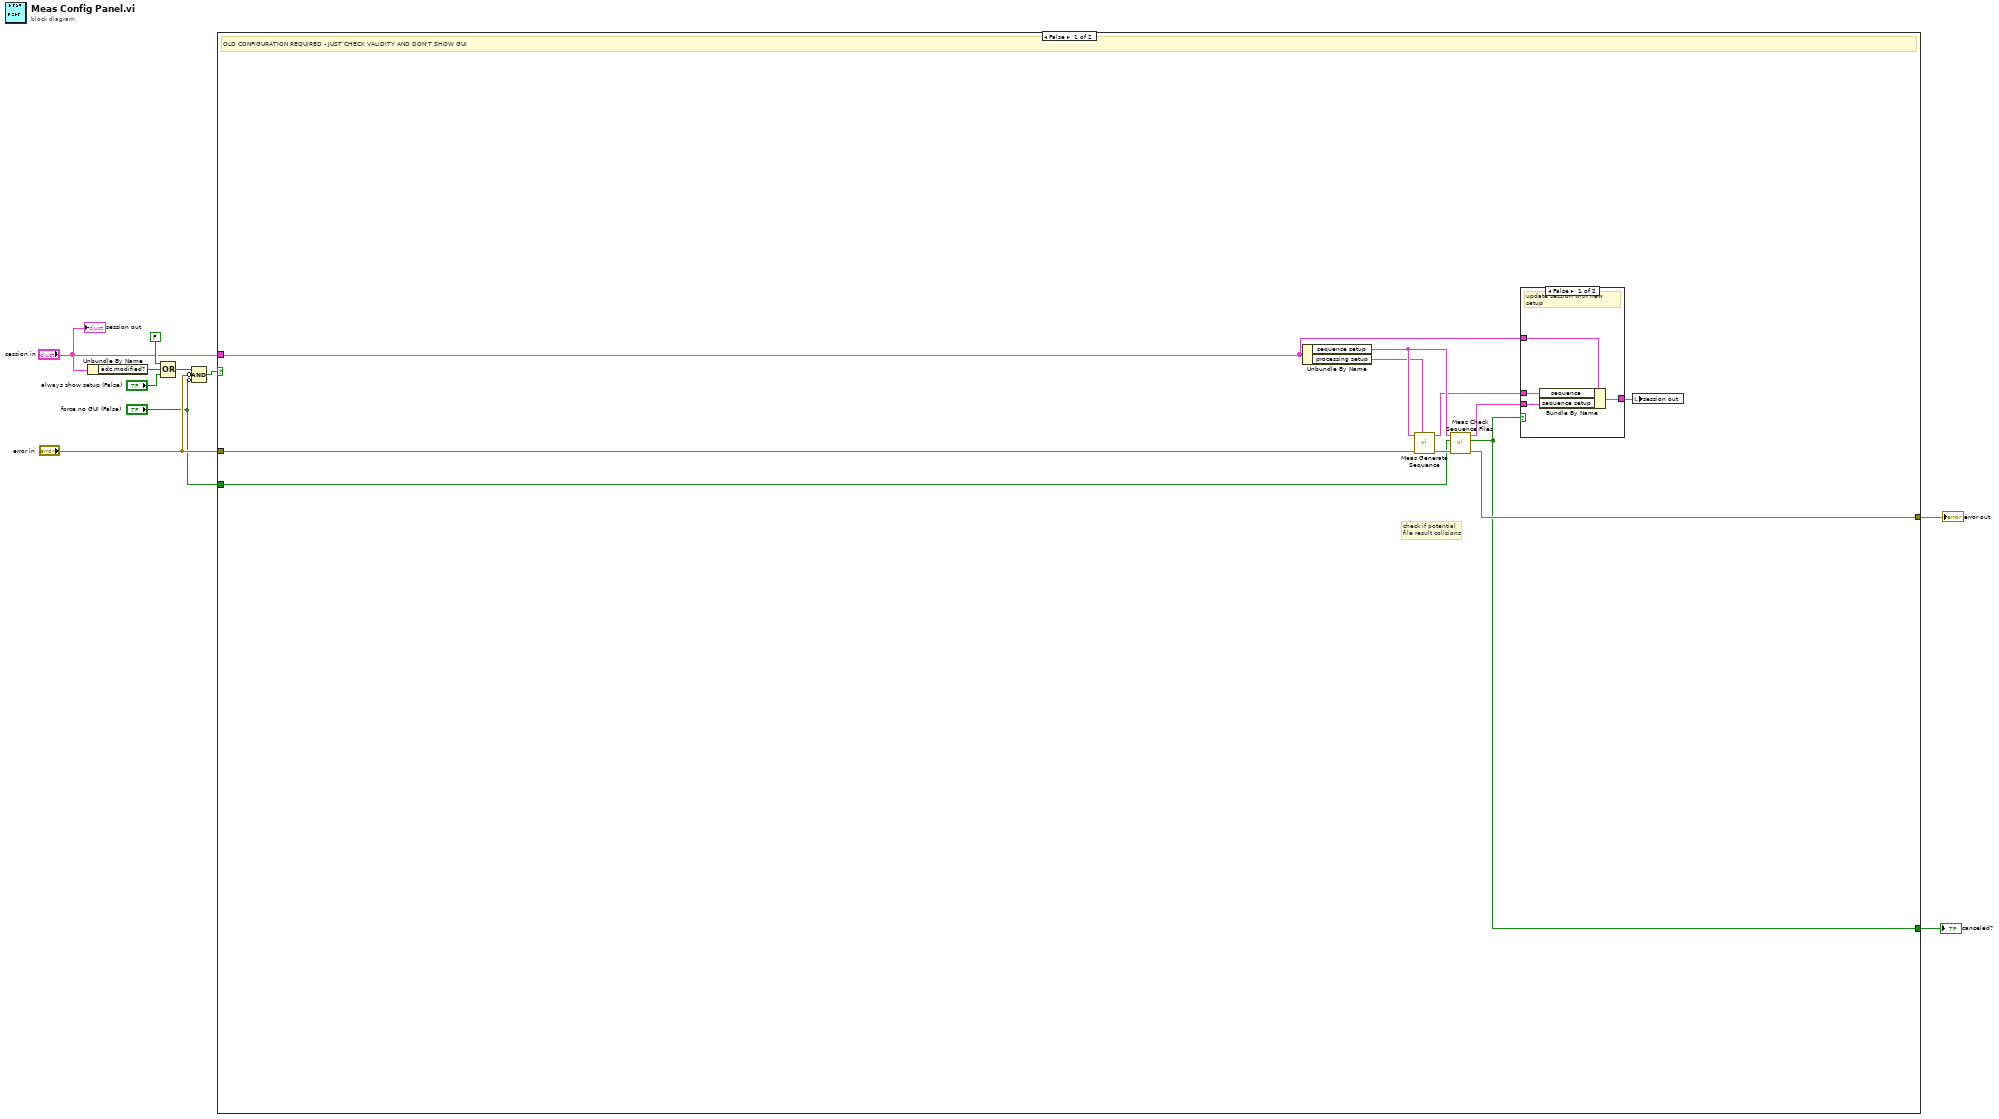
[diagram p0: block diagram]
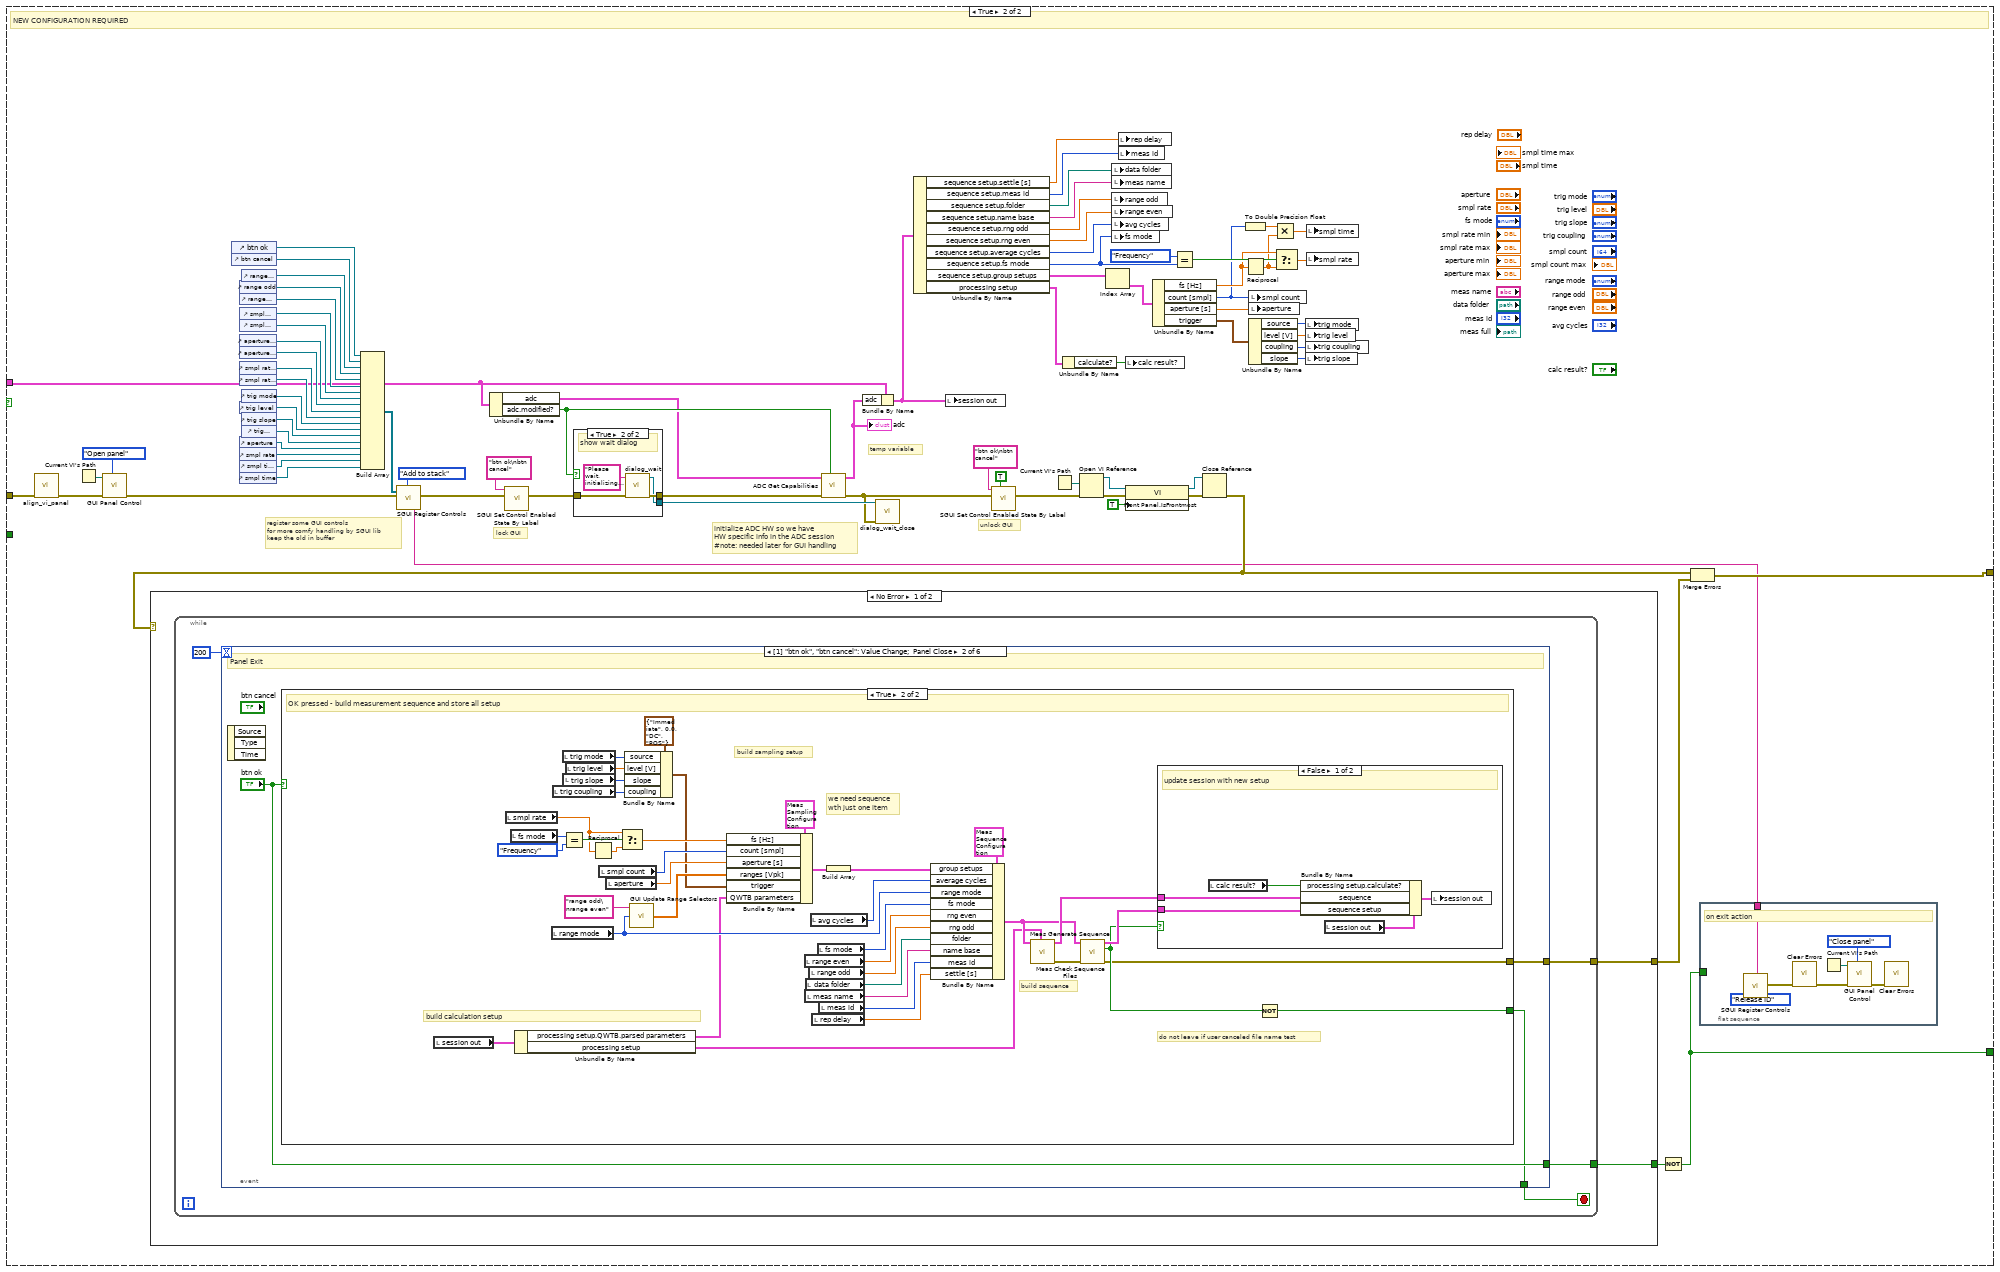
[diagram p3: hidden frame]
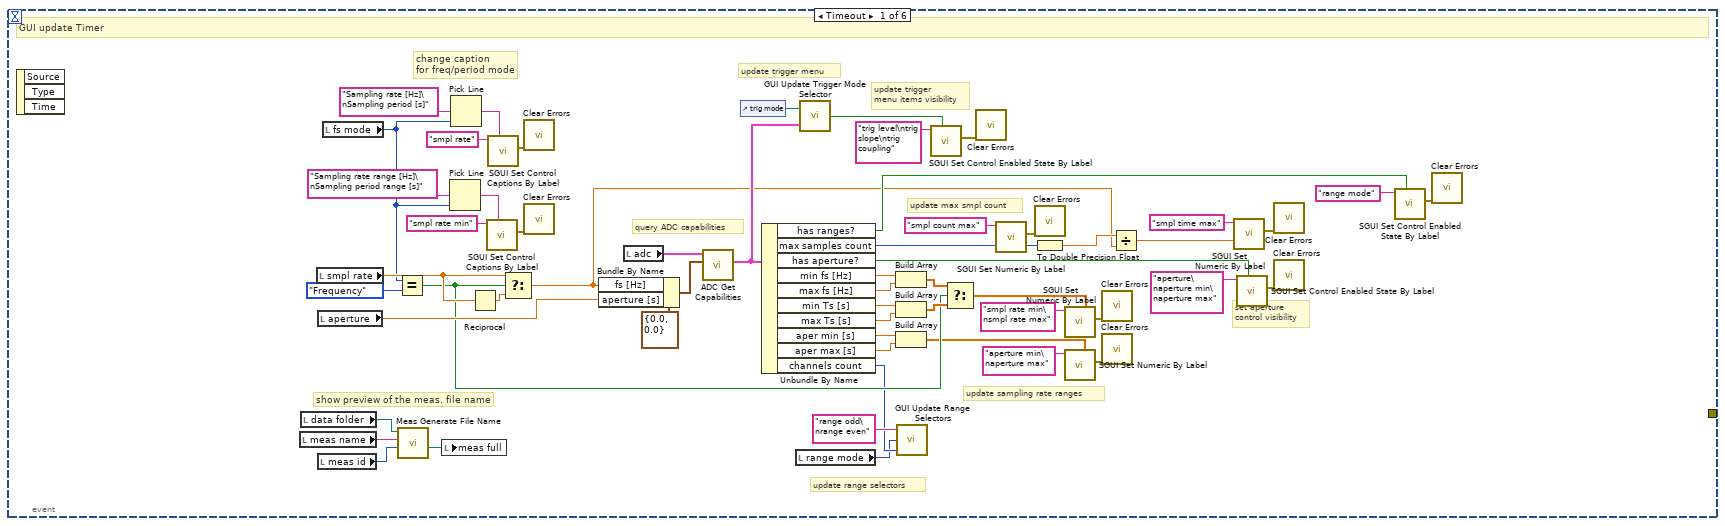
[diagram p5: hidden frame]
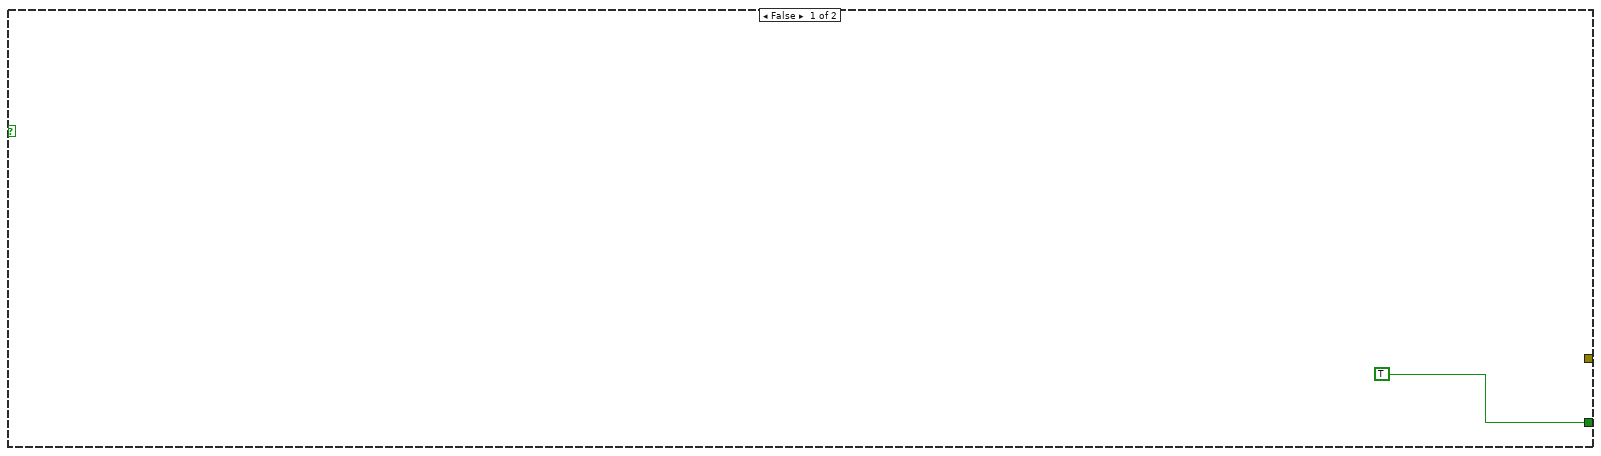
[diagram p6: hidden frame]
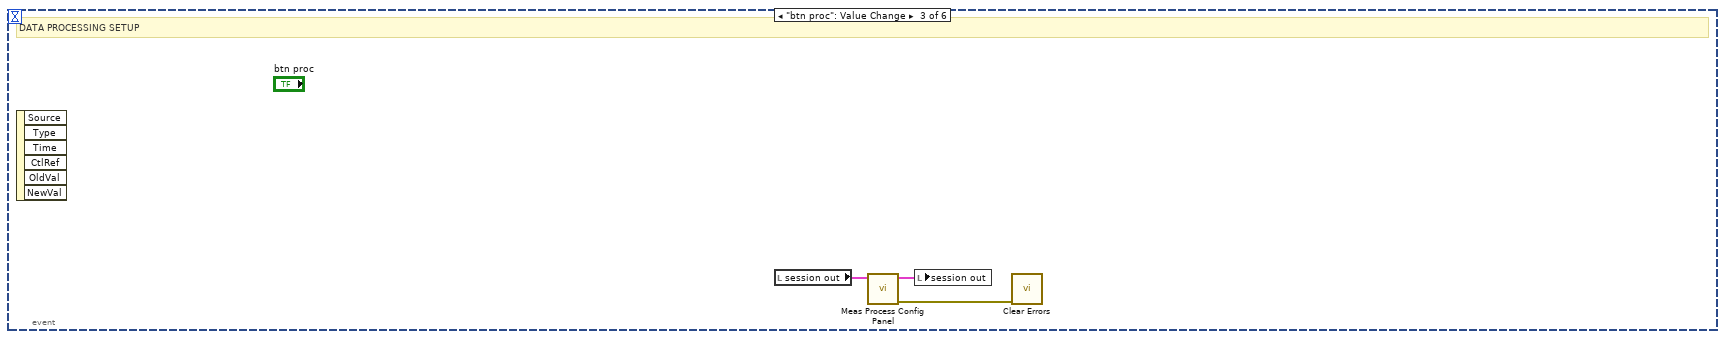
[diagram p8: hidden frame]
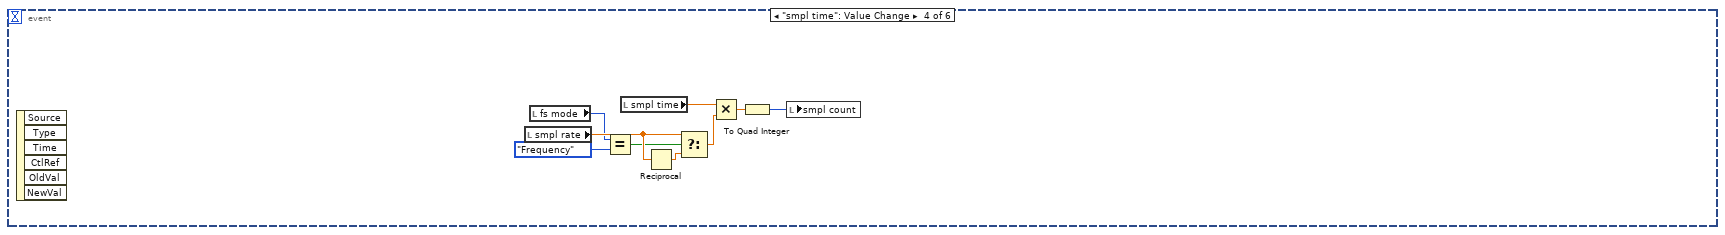
[diagram p9: hidden frame]
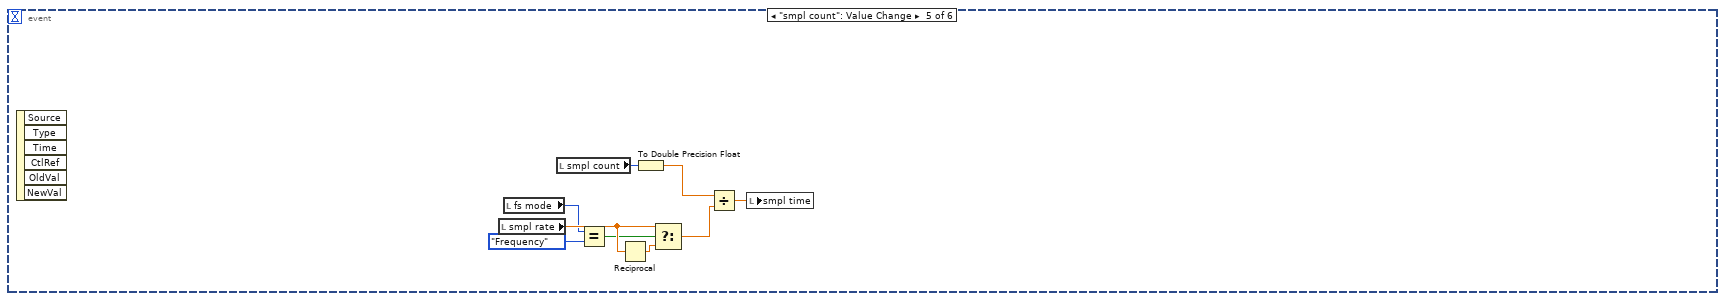
[diagram p10: hidden frame]
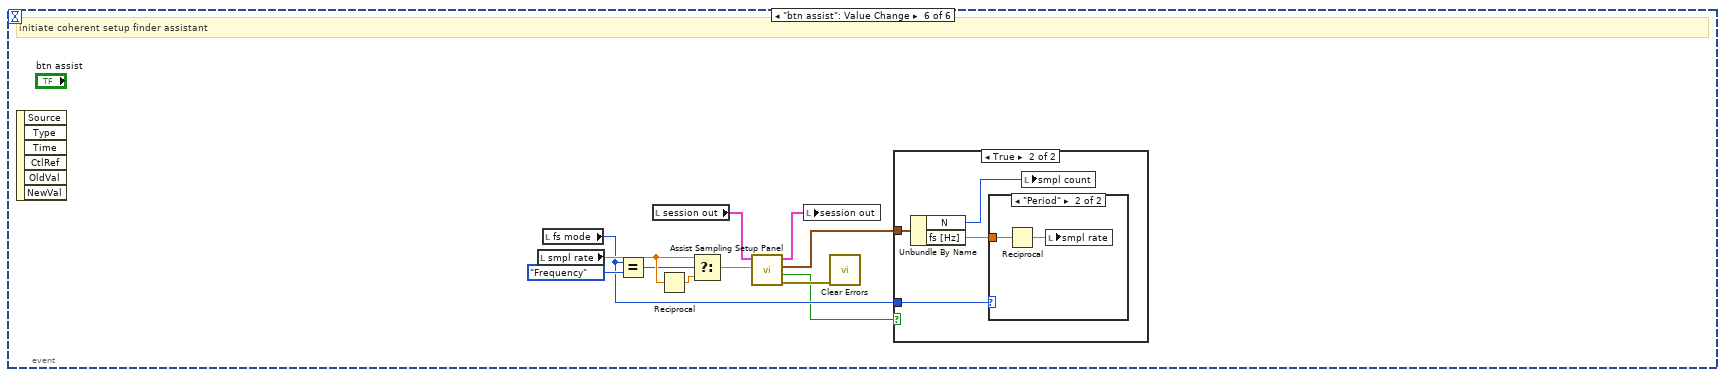
[diagram p11: hidden frame]
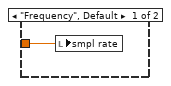
[diagram p13: hidden frame]
diagram:
  n1 = Unbundle By Name("session in") -> ("adc.modified?"=w9:bool)
  n2 = Compound Arithmetic op=OR(FALSE ("value"), w9, "always show setup (False)") -> (w7:bool)
  n3 = Compound Arithmetic op=AND(w7, invert "error in", invert "force no GUI (False)") -> (w10:bool)
  n4 = case shown="False" w10 {
    tunnel: "error in" -> [w20 w57]
    tunnel: "session in" -> [w12 w49]
    tunnel: [w16 w41] -> w4
    tunnel: [w21 w31] -> w3
    tunnel: "force no GUI (False)" -> [w13 _]
    frame False {
      # "check if potential\nfile result colisions"
      # "OLD CONFIGURATION REQUIRED - JUST CHECK VALIDITY AND DON'T SHOW GUI"
      n5 = Unbundle By Name(w12) -> ("sequence setup"=w18:T53, "processing setup"=w17:T55)
      n6 = call "Meas Generate Sequence.vi"("processing setup"=w17, "error in"=w20, "sequence setup"=w18) -> ("error out"=w19:errorcluster, "sequence out"=w15:T49[])  [unwired: 6 in, 1 out]
      n7 = call "Meas Check Sequence Files.vi"("error in"=w19, "don't ask (False)"=w13, "sequence setup"=w18) -> ("error out"=w21:errorcluster, "cancel?"=w16:bool, "sequence setup out (copy)"=w14:T53)  [unwired: 6 in]
      n8 = case shown="False" w16 {
        tunnel: w15 -> [w25 _]
        tunnel: w14 -> [w24 _]
        tunnel: w12 -> [w23 w26]
        tunnel: [w22 w26] -> w11
        frame False {
          # "update session with new setup"
          n9 = Bundle By Name(cluster=w23, "sequence"=w25, "sequence setup"=w24) -> (w22:T48)
        }
        frame True {
        }
      }
      n10 = local write "session out"(w11) -> ()
    }
    frame True {
      # "unlock GUI"
      # "lock GUI"
      # "temp variable"
      # "register some GUI controls\nfor more comfy handling by SGUI lib\nkeep the old in buffer"
      # "initialize ADC HW so we have\nHW specific info in the ADC session\n#note: needed later for GUI handling"
      # "NEW CONFIGURATION REQUIRED"
      n11 = call "align_vi_panel.vi"("error in"=w57) -> ("error out"=w46:errorcluster)  [unwired: 10 in]
      n12 = Current VI's Path() -> (path=w44:path)
      n13 = call "GUI Panel Control.vi"("action (open panel)"=GUI_Panel_Control_Action."Open panel", "error in (no error)"=w46, "vi path"=w44) -> ("error out"=w45:errorcluster)  [unwired: 8 in]
      n14 = control-ref of="btn ok"() -> (w66:refnum<vi>)
      n15 = control-ref of="btn cancel"() -> (w67:refnum<vi>)
      n16 = control-ref of="range odd"() -> (w90:refnum<vi>)
      n17 = control-ref of="range even"() -> (w89:refnum<vi>)
      n18 = control-ref of="smpl count"() -> (w91:refnum<vi>)
      n19 = control-ref of="smpl count max"() -> (w92:refnum<vi>)
      n20 = control-ref of="aperture min"() -> (w94:refnum<vi>)
      n21 = control-ref of="aperture max"() -> (w93:refnum<vi>)
      n22 = control-ref of="smpl rate min"() -> (w95:refnum<vi>)
      n23 = control-ref of="smpl rate max"() -> (w96:refnum<vi>)
      n24 = control-ref of="trig level"() -> (w98:refnum<vi>)
      n25 = control-ref of="aperture"() -> (w101:refnum<vi>)
      n26 = control-ref of="smpl rate"() -> (w103:refnum<vi>)
      n27 = control-ref of="smpl time max"() -> (w35:refnum<vi>)
      n28 = control-ref of="smpl time"() -> (w34:refnum<vi>)
      n29 = control-ref of="range mode"() -> (w68:refnum<vi>)
      n30 = control-ref of="trig mode"() -> (w97:refnum<vi>)
      n31 = control-ref of="trig slope"() -> (w99:refnum<vi>)
      n32 = control-ref of="trig coupling"() -> (w100:refnum<vi>)
      n33 = Build Array(w66, w67, w68, w90, w89, w91, w92, w94, w93, w95, w96, w97, w98, w99, w100, w101, w103, w35, w34) -> (w104:refnum<vi>[])
      n34 = call "SGUI Register Controls.vi"("error in"=w45, "control references (empty)"=w104, "register mode (overwrite)"=SGUI_Assign_References_Mode."Add to stack") -> ("assigned ID"=w30:string, "error out"=w65:errorcluster)  [unwired: 14 in, 1 out]
      n35 = Unbundle By Name(w49) -> ("adc"=w28:T5, "adc.modified?"=w62:bool)
      n36 = call "SGUI Set Control Enabled State By Label.vi"("error in"=w65, "labels (empty)"="btn ok\nbtn cancel") -> ("error out"=w63:errorcluster)  [unwired: 8 in, 1 out]
      n37 = case shown="True" w62 {
        tunnel: w63 -> [w105 w109]
        tunnel: [w105 w108] -> w29
        tunnel: [_ w106] -> w61
        frame False {
        }
        frame True {
          # "show wait dialog"
          n38 = call "dialog_wait.vi"("error in"=w109, "message string"="Please wait, initializing HW ...") -> ("error out"=w108:errorcluster, "reference out"=w106:refnum<vi>)  [unwired: 8 in]
        }
      }
      n39 = call "ADC Get Capabilities.vi"("Initialize HW? (False)"=w62, "error in"=w29, "adc session in"=w28) -> ("error out"=w60:errorcluster, "adc session out"=w102:T5)  [unwired: 6 in, 1 out]
      "adc" <- w102
      n40 = Bundle By Name(cluster=w49, "adc"=w102) -> (w40:T48)
      n41 = call "dialog_wait_close.vi"("error in"=w60, "async vi ref"=w61) -> ()  [unwired: 2 in]
      n42 = Unbundle By Name(w40) -> ("sequence setup.settle [s]"=w27:dbl, "sequence setup.meas id"=w42:i32, "sequence setup.folder"=w70:path, "sequence setup.name base"=w71:string, "sequence setup.rng odd"=w72:dbl, "sequence setup.rng even"=w73:dbl, "sequence setup.average cycles"=w83:i32, "sequence setup.fs mode"=w81:T47, "sequence setup.group setups"=w87:T50[], "processing setup"=w51:T55)
      n43 = local write "session out"(w40) -> ()
      n44 = call "SGUI Set Control Enabled State By Label.vi"("error in"=w60, "labels (empty)"="btn ok\nbtn cancel", "Enabled? (False)"=TRUE) -> ("error out"=w53:errorcluster)  [unwired: 7 in, 1 out]
      n45 = Current VI's Path() -> (path=w56:path)
      n46 = Unbundle By Name(w51) -> ("calculate?"=w50:bool)
      n47 = Open VI Reference(vi path=w56, error in (no error)=w53) -> (vi reference=w55:refnum<vi>, error out=w54:errorcluster)  [unwired: 4 in]
      n48 = Index Array(array=w87) -> (element=w86:T50)  [unwired: 1 in]
      n49 = local write "data folder"(w70) -> ()
      n50 = local write "meas name"(w71) -> ()
      n51 = local write "range odd"(w72) -> ()
      n52 = local write "range even"(w73) -> ()
      n53 = local write "avg cycles"(w83) -> ()
      n54 = local write "fs mode"(w81) -> ()
      n55 = local write "rep delay"(w27) -> ()
      n56 = local write "meas id"(w42) -> ()
      n57 = local write "calc result?"(w50) -> ()
      n58 = property class="VI"(reference=w55, error in=w54, "Front Panel.IsFrontmost"=TRUE ("Front Panel Window:Is Frontmost")) -> (reference out=w47:refnum<vi>, error out=w48:errorcluster)
      n59 = Unbundle By Name(w86) -> ("fs [Hz]"=w84:dbl, "count [smpl]"=w36:i64, "aperture [s]"=w79:dbl, "trigger"=w78:T51)
      n60 = Equal?(x=Meas_Sampling_Rate_Mode."Frequency", y=w81) -> (x = y?=w85:bool)
      n61 = Close Reference(reference=w47, error in (no error)=w48) -> (error out=w33:errorcluster)
      n62 = case shown="No Error" w33 {
        tunnel: [w118 _] -> w88
        tunnel: [w117 _] -> w32
        frame No Error {
          n63 = while {
            tunnel: [w120] -> w118
            tunnel: [w119] -> w117
            stop <- w121 stop-if-true
            n64 = event shown="[1] \"btn ok\", \"btn cancel\": Value Change;  Panel Close" {
              selector: _ -> [_ _ _ _ _ _]
              dyn-events: _ -> [_ _ _ _ _ _]
              timeout: 200 -> [_ _ _ _ _ _]
              tunnel: [_ w181 _ _ _ _] -> w121
              tunnel: [_ "btn ok" _ _ _ _] -> w120
              tunnel: [_ w180 _ _ _ _] -> w119
              event Timeout {
                # "show preview of the meas. file name"
                # "update range selectors"
                # "update sampling rate ranges"
                # "update max smpl count"
                # "update trigger\nmenu items visibility"
                # "update trigger menu"
                # "set aperture\ncontrol visibility"
                # "query ADC capabilities"
                # "change caption\nfor freq/period mode"
                # "GUI update Timer"
                n65 = event-data() -> ()  [unwired: 1 in, 3 out]
                n66 = local read "meas name"() -> (w132:string)
                n67 = local read "data folder"() -> (w130:path)
                n68 = local read "smpl rate"() -> (w172:dbl)
                n69 = local read "aperture"() -> (w168:dbl)
                n70 = local read "meas id"() -> (w131:i32)
                n71 = local read "fs mode"() -> (w153:T47)
                n72 = Equal?(x=w153, y=Meas_Sampling_Rate_Mode."Frequency") -> (x = y?=w157:bool)
                n73 = call "Meas Generate File Name.vi"("meas id"=w131, "name base"=w132, "folder"=w130) -> ("header file full path"=w129:path)  [unwired: 4 in, 4 out]
                n74 = local write "meas full"(w129) -> ()
                n75 = Pick Line(multi-line string="Sampling rate range [Hz]\nSampling period range [s]", line index=w153) -> (output string=w155:string)  [unwired: 1 in]
                n76 = Pick Line(multi-line string="Sampling rate [Hz]\nSampling period [s]", line index=w153) -> (output string=w177:string)  [unwired: 1 in]
                n77 = Reciprocal(x=w172) -> (1/x=w171:dbl)
                n78 = call "SGUI Set Control Captions By Label.vi"("labels (empty)"="smpl rate min", "captions (empty)"=w155) -> ("error out"=w139:errorcluster)  [unwired: 8 in, 1 out]
                n79 = call "SGUI Set Control Captions By Label.vi"("labels (empty)"="smpl rate", "captions (empty)"=w177) -> ("error out"=w140:errorcluster)  [unwired: 8 in, 1 out]
                n80 = Select(t=w172, s=w157, f=w171) -> (s? t:f=w123:dbl)
                n81 = call <vilib>:"Clear Errors.vi"("error in (no error)"=w140) -> ()  [unwired: 6 in, 1 out]
                n82 = call <vilib>:"Clear Errors.vi"("error in (no error)"=w139) -> ()  [unwired: 6 in, 1 out]
                n83 = Bundle By Name(cluster=T69 {"fs [Hz]"=0.0, "aperture [s]"=0.0} ("parameters"), "fs [Hz]"=w123, "aperture [s]"=w168) -> (w174:T69)
                n84 = local read "adc"() -> (w176:T5)
                n85 = call "ADC Get Capabilities.vi"("parameters"=w174, "adc session in"=w176) -> ("capabilities"=w167:T70)  [unwired: 7 in, 2 out]
                n86 = control-ref of="trig mode"() -> (w166:refnum<vi>)
                n87 = Unbundle By Name(w167) -> ("has ranges?"=w133:bool, "max samples count"=w128:i64, "has aperture?"=w169:bool, "min fs [Hz]"=w163:ext, "max fs [Hz]"=w162:ext, "min Ts [s]"=w161:ext, "max Ts [s]"=w160:ext, "aper min [s]"=w150:dbl, "aper max [s]"=w149:dbl, "channels count"=w137:i32)
                n88 = local read "range mode"() -> (w136:T1)
                n89 = call "GUI Update Trigger Mode Selector.vi"("capabilities"=w167, "trig mode ref"=w166) -> ("has parameters?"=w164:bool)
                n90 = Build Array(w163, w162) -> (w159:ext[])
                n91 = Build Array(w161, w160) -> (w158:ext[])
                n92 = Build Array(w150, w149) -> (w147:dbl[])
                n93 = call "GUI Update Range Selectors.vi"("total channels"=w137, "range mode"=w136, "odd and even item names"="range odd\nrange even") -> ()  [unwired: 1 out]
                n94 = call "SGUI Set Control Enabled State By Label.vi"("labels (empty)"="trig level\ntrig slope\ntrig coupling", "Enabled? (False)"=w164) -> ("error out"=w145:errorcluster)  [unwired: 8 in, 1 out]
                n95 = Select(t=w159, s=w157, f=w158) -> (s? t:f=w152:ext[])
                n96 = call <vilib>:"Clear Errors.vi"("error in (no error)"=w145) -> ()  [unwired: 6 in, 1 out]
                n97 = call-poly "SGUI Set Numeric By Label.vi"("label (empty)"="smpl count max" ("labels (empty)"), "value (none)"=w128) -> ("error out"=w144:errorcluster)  [unwired: 8 in, 1 out]
                n98 = call <vilib>:"Clear Errors.vi"("error in (no error)"=w144) -> ()  [unwired: 6 in, 1 out]
                n99 = To Double Precision Float(number=w128) -> (double precision float=w124:dbl)
                n100 = call-poly "SGUI Set Numeric By Label.vi"("labels (empty)"="smpl rate min\nsmpl rate max", "numbers (empty)"=w152) -> ("error out"=w143:errorcluster)  [unwired: 8 in, 1 out]
                n101 = call-poly "SGUI Set Numeric By Label.vi"("labels (empty)"="aperture min\naperture max", "numbers (empty)"=w147) -> ("error out"=w142:errorcluster)  [unwired: 8 in, 1 out]
                n102 = call <vilib>:"Clear Errors.vi"("error in (no error)"=w143) -> ()  [unwired: 6 in, 1 out]
                n103 = call <vilib>:"Clear Errors.vi"("error in (no error)"=w142) -> ()  [unwired: 6 in, 1 out]
                n104 = Divide(x=w124, y=w123) -> (x/y=w127:dbl)
                n105 = call-poly "SGUI Set Numeric By Label.vi"("label (empty)"="smpl time max", "value (none)"=w127) -> ("error out"=w125:errorcluster)  [unwired: 8 in, 1 out]
                n106 = call "SGUI Set Control Enabled State By Label.vi"("labels (empty)"="aperture\naperture min\naperture max", "Enabled? (False)"=w169) -> ("error out"=w141:errorcluster)  [unwired: 8 in, 1 out]
                n107 = call <vilib>:"Clear Errors.vi"("error in (no error)"=w125) -> ()  [unwired: 6 in, 1 out]
                n108 = call <vilib>:"Clear Errors.vi"("error in (no error)"=w141) -> ()  [unwired: 6 in, 1 out]
                n109 = call "SGUI Set Control Enabled State By Label.vi"("labels (empty)"="range mode", "Enabled? (False)"=w133) -> ("error out"=w135:errorcluster)  [unwired: 8 in, 1 out]
                n110 = call <vilib>:"Clear Errors.vi"("error in (no error)"=w135) -> ()  [unwired: 6 in, 1 out]
              }
              event "btn ok", "btn cancel": Value Change; Panel Close {
                # "Panel Exit"
                n111 = event-data() -> ()  [unwired: 1 in, 3 out]
                n112 = case shown="True" "btn ok" {
                  tunnel: [TRUE w190] -> w181
                  tunnel: [_ w185] -> w180
                  frame False {
                  }
                  frame True {
                    # "build calculation setup"
                    # "do not leave if user canceled file name test"
                    # "build sequence"
                    # "we need sequence\nwth just one item"
                    # "build sampling setup"
                    # "OK pressed - build measurement sequence and store all setup"
                    n113 = local read "session out"() -> (w188:T48)
                    n114 = local read "smpl rate"() -> (w218:dbl)
                    n115 = local read "fs mode"() -> (w221:T47)
                    n116 = Unbundle By Name(w188) -> ("processing setup.QWTB.parsed parameters"=w187:T52[], "processing setup"=w186:T55)
                    n117 = local read "range mode"() -> (w203:T1)
                    n118 = local read "trig coupling"() -> (w209:T2)
                    n119 = local read "trig mode"() -> (w206:T4)
                    n120 = Equal?(x=w221, y=Meas_Sampling_Rate_Mode."Frequency") -> (x = y?=w219:bool)
                    n121 = local read "trig slope"() -> (w208:T3)
                    n122 = local read "trig level"() -> (w207:dbl)
                    n123 = Reciprocal(x=w218) -> (1/x=w217:dbl)
                    n124 = local read "smpl count"() -> (w215:i64)
                    n125 = local read "aperture"() -> (w214:dbl)
                    n126 = Select(t=w218, s=w219, f=w217) -> (s? t:f=w216:dbl)
                    n127 = Bundle By Name(cluster=T51 {"source"=enum."Immediate", "level [V]"=0.0, "coupling"=enum."DC", "slope"=enum."POS"} ("trigger"), "source"=w206, "level [V]"=w207, "slope"=w208, "coupling"=w209) -> (w210:T51)
                    n128 = call "GUI Update Range Selectors.vi"("range mode"=w203, "odd and even item names"="range odd\nrange even") -> ("ranges vector [V]"=w212:dbl[])  [unwired: 1 in]
                    n129 = Bundle By Name(cluster=T50 {"fs [Hz]"=0.0, "count [smpl]"=0, "aperture [s]"=0.0, "trigger"={"source"=enum."Immediate", "level [V]"=0.0, "coupling"=enum."DC", "slope"=enum."POS"}, "ranges [Vpk]"=[], "QWTB parameters"=[]} ("meas config"), "fs [Hz]"=w216, "count [smpl]"=w215, "aperture [s]"=w214, "ranges [Vpk]"=w212, "trigger"=w210, "QWTB parameters"=w187) -> (w205:T50)
                    n130 = local read "range even"() -> (w201:dbl)
                    n131 = local read "meas name"() -> (w198:string)
                    n132 = local read "data folder"() -> (w199:path)
                    n133 = local read "range odd"() -> (w200:dbl)
                    n134 = local read "avg cycles"() -> (w196:i32)
                    n135 = local read "rep delay"() -> (w184:dbl)
                    n136 = local read "fs mode"() -> (w202:T47)
                    n137 = local read "meas id"() -> (w189:i32)
                    n138 = Build Array(w205) -> (w197:T50[])
                    n139 = Bundle By Name(cluster=T53 {"group setups"=[], "average cycles"=0, "range mode"=enum."Keep defaults", "fs mode"=enum."Frequency", "rng even"=0.0, "rng odd"=0.0, "folder"=path "", "name base"="", "meas id"=0, "settle [s]"=0.0} ("sequence setup"), "group setups"=w197, "average cycles"=w196, "range mode"=w203, "fs mode"=w202, "rng even"=w201, "rng odd"=w200, "folder"=w199, "name base"=w198, "meas id"=w189, "settle [s]"=w184) -> (w193:T53)
                    n140 = call "Meas Generate Sequence.vi"("processing setup"=w186, "sequence setup"=w193) -> ("error out"=w195:errorcluster, "sequence out"=w194:T49[])  [unwired: 7 in, 1 out]
                    n141 = call "Meas Check Sequence Files.vi"("error in"=w195, "sequence setup"=w193) -> ("error out"=w185:errorcluster, "cancel?"=w191:bool, "sequence setup out (copy)"=w192:T53)  [unwired: 7 in]
                    n142 = case shown="False" w191 {
                      tunnel: w194 -> [w225 _]
                      tunnel: w192 -> [w224 _]
                      frame False {
                        # "update session with new setup"
                        n143 = local read "calc result?"() -> (w223:bool)
                        n144 = local read "session out"() -> (w227:T48)
                        n145 = Bundle By Name(cluster=w227, "processing setup.calculate?"=w223, "sequence"=w225, "sequence setup"=w224) -> (w226:T48)
                        n146 = local write "session out"(w226) -> ()
                      }
                      frame True {
                      }
                    }
                    n147 = Not(x=w191) -> (.not. x?=w190:bool)
                  }
                }
              }
              event "btn proc": Value Change {
                # "DATA PROCESSING SETUP"
                n148 = event-data() -> ()  [unwired: 1 in, 6 out]
                n149 = local read "session out"() -> (w230:T48)
                n150 = call "Meas Process Config Panel.vi"("session in"=w230) -> ("error out"=w228:errorcluster, "session out"=w229:T48)  [unwired: 9 in]
                n151 = local write "session out"(w229) -> ()
                n152 = call <vilib>:"Clear Errors.vi"("error in (no error)"=w228) -> ()  [unwired: 6 in, 1 out]
              }
              event "smpl time": Value Change {
                n153 = event-data() -> ()  [unwired: 1 in, 6 out]
                n154 = local read "smpl rate"() -> (w238:dbl)
                n155 = local read "fs mode"() -> (w235:T47)
                n156 = Equal?(x=w235, y=Meas_Sampling_Rate_Mode."Frequency") -> (x = y?=w236:bool)
                n157 = local read "smpl time"() -> (w234:dbl)
                n158 = Reciprocal(x=w238) -> (1/x=w237:dbl)
                n159 = Select(t=w238, s=w236, f=w237) -> (s? t:f=w233:dbl)
                n160 = Multiply(x=w234, y=w233) -> (x*y=w232:dbl)
                n161 = To Quad Integer(1:w232) -> (0:w231:i64)
                n162 = local write "smpl count"(w231) -> ()
              }
              event "smpl count": Value Change {
                n163 = event-data() -> ()  [unwired: 1 in, 6 out]
                n164 = local read "smpl rate"() -> (w247:dbl)
                n165 = local read "fs mode"() -> (w244:T47)
                n166 = local read "smpl count"() -> (w243:i64)
                n167 = Equal?(x=w244, y=Meas_Sampling_Rate_Mode."Frequency") -> (x = y?=w245:bool)
                n168 = Reciprocal(x=w247) -> (1/x=w246:dbl)
                n169 = To Double Precision Float(number=w243) -> (double precision float=w242:dbl)
                n170 = Select(t=w247, s=w245, f=w246) -> (s? t:f=w241:dbl)
                n171 = Divide(x=w242, y=w241) -> (x/y=w240:dbl)
                n172 = local write "smpl time"(w240) -> ()
              }
              event "btn assist": Value Change {
                # "initiate coherent setup finder assistant"
                n173 = event-data() -> ()  [unwired: 1 in, 6 out]
                n174 = local read "smpl rate"() -> (w257:dbl)
                n175 = local read "fs mode"() -> (w250:T47)
                n176 = Equal?(x=w250, y=Meas_Sampling_Rate_Mode."Frequency") -> (x = y?=w255:bool)
                n177 = local read "session out"() -> (w253:T48)
                n178 = Reciprocal(x=w257) -> (1/x=w256:dbl)
                n179 = Select(t=w257, s=w255, f=w256) -> (s? t:f=w254:dbl)
                n180 = call "Assist Sampling Setup Panel.vi"("fs in [Hz]"=w254, "session in"=w253) -> ("error out"=w259:errorcluster, "ok"=w249:bool, "smpl setup"=w251:T72, "session out"=w252:T48)  [unwired: 6 in]
                n181 = local write "session out"(w252) -> ()
                n182 = call <vilib>:"Clear Errors.vi"("error in (no error)"=w259) -> ()  [unwired: 6 in, 1 out]
                n183 = case shown="True" w249 {
                  tunnel: w251 -> [_ w263]
                  tunnel: w250 -> [_ w262]
                  frame False {
                  }
                  frame True {
                    n184 = Unbundle By Name(w263) -> ("N"=w260:i64, "fs [Hz]"=w261:ext)
                    n185 = case shown="\"Period\"" w262 {
                      tunnel: w261 -> [w264 w266]
                      frame "Frequency", Default {
                        n186 = local write "smpl rate"(w264) -> ()
                      }
                      frame "Period" {
                        n187 = Reciprocal(x=w266) -> (1/x=w265:ext)
                        n188 = local write "smpl rate"(w265) -> ()
                      }
                    }
                    n189 = local write "smpl count"(w260) -> ()
                  }
                }
              }
            }
          }
        }
        frame Error {
        }
      }
      n190 = To Double Precision Float(number=w36) -> (double precision float=w38:dbl)
      n191 = Reciprocal(x=w84) -> (1/x=w39:dbl)
      n192 = local write "smpl count"(w36) -> ()
      n193 = local write "aperture"(w79) -> ()
      n194 = Unbundle By Name(w78) -> ("source"=w77:T4, "level [V]"=w76:dbl, "coupling"=w75:T2, "slope"=w74:T3)
      n195 = Multiply(x=w38, y=w39) -> (x*y=w37:dbl)
      n196 = Select(t=w84, s=w85, f=w39) -> (s? t:f=w80:dbl)
      n197 = local write "trig mode"(w77) -> ()
      n198 = local write "trig level"(w76) -> ()
      n199 = local write "trig coupling"(w75) -> ()
      n200 = local write "trig slope"(w74) -> ()
      n201 = local write "smpl time"(w37) -> ()
      n202 = local write "smpl rate"(w80) -> ()
      n203 = Not(x=w88) -> (.not. x?=w41:bool)
      n204 = Merge Errors(w33, w32) -> (w31:errorcluster)
      n205 = flat-sequence {
        tunnel: w41 -> [_]
        tunnel: w30 -> [w110]
        frame #0 {
          # "on exit action"
          n206 = call "SGUI Register Controls.vi"("register mode (overwrite)"=SGUI_Assign_References_Mode."Release ID", "controls ID (empty)"=w110) -> ("error out"=w115:errorcluster)  [unwired: 15 in, 2 out]
          n207 = call <vilib>:"Clear Errors.vi"("error in (no error)"=w115) -> ("error out"=w112:errorcluster)  [unwired: 6 in]
          n208 = Current VI's Path() -> (path=w114:path)
          n209 = call "GUI Panel Control.vi"("action (open panel)"=GUI_Panel_Control_Action."Close panel", "error in (no error)"=w112, "vi path"=w114) -> ("error out"=w111:errorcluster)  [unwired: 8 in]
          n210 = call <vilib>:"Clear Errors.vi"("error in (no error)"=w111) -> ()  [unwired: 6 in, 1 out]
        }
      }
    }
  }
  "canceled?" <- w4
  "error out" <- w3
  "session out" <- "session in"
